vi "gyro-V2.vi"() -> ()   [LabVIEW 2016]
uses:
  lorentzian.ctl
  circle corners.ctl
  <vilib>/event_ctls.llb/eventvkey.ctl
  peak -- parameters -- complex fit.ctl
  wavepacket.ctl
  filter method control.ctl
  cursor winow.ctl
  parameters -- scan monitor control.ctl
  pid -- parameters.ctl
  agregator -- action.ctl
  plot refs -- filter related.ctl
  MFLI controller action.ctl
  cursor window action.ctl
  sweep parameters.ctl
  cursor action.ctl
  KM_file -- read-write control.ctl
  linear interpolation - real.vi
  linear interpolation iiii- complex.vi
  aggregator - v - real - atomic.vi
  Q - not nan -- real.vi
  filter - complex - four.vi
  linear interp iiii- complex - z-omega.vi
  peak -- PM find lorenzian - V3.vi
  tale of three indices.vi
  filter -- window span logic.vi
  linear interp iiii- complex - z-omega - divide.vi
  containing bix.vi
  <vilib>/Analysis/baseanly.llb/A x B.vi
  <vilib>/Analysis/baseanly.llb/Complex A x B.vi
  line -- complex.vi
  Q -- check range -- i -- integer.vi
  peak -- guess at omega -- dzdomega V2.vi
  command stack.vi
  tale of three indices -- check state.vi
  Q - not nan -- integer.vi
  peak -- z center from mult phase points.vi
  peak -- estimate for lorentzian.vi
  peak -- fake phase around center.vi
  peak -- get weights.vi
  peak -- four corner circle transformation logic.vi
  peak - fit phase around center - V2.vi
  array - generate range.vi
  circle center from three points.vi
  <vilib>/Utility/error.llb/Clear Errors.vi
  peak -- fit function -- minus arctan.vi
  <vilib>/Analysis/Matrix/Numeric/Conversions/Array To Matrix.vi
  <vilib>/Analysis/Matrix/Numeric/Conversions/Array To Matrix - RA2.vi
  <vilib>/Analysis/baseanly.llb/Inverse Matrix.vi
  <vilib>/Analysis/baseanly.llb/Real Inverse Matrix.vi
  <vilib>/gmath/NumericalOptimization/Nonlinear Curve Fit.vi
  <vilib>/gmath/NumericalOptimization/Nonlinear Curve Fit LM.vi
  KM_filter pipe - plot staff - more - V3.vi
  four-corner circle transformation.ctl
panel:
  in  "all":enum32{"all", "other"}(tab)
  out "angle (deg)":dbl=1994442.711851292 format="%#11_11f"
  out "Temperature (K)":dbl=1994442.711851292 format="%#11_11f"
  out "Field (T)":dbl=1994442.711851292 format="%#11_11f"
  out "Plot: circle sweep window":cluster{"all rows":dbl[], "all rows":dbl[]}[](graph)=[{"all rows"=[1907168.346185415, 1965249.3711735276, 1976970.6285003964, 1982011.816659579, 1984821.3372776513, 1986615.362944235, 1987862.2368974418, 1988780.6904674931, 1989486.5864630162, 1990047.0317770669, 1990503.5833778584, 1990883.3521453317, 1991204.7790270294, 1991480.8449781418, 1991720.9531195113, 1991932.0825617604, 1992119.5227900057, 1992287.356339517, 1992438.7849751213, 1992576.3555406206, 1992702.1197279515, 1992817.749276128, 1992924.6204638672, 1993023.8770414377, 1993116.4777602106, 1993203.2327275807, 1993284.831541473, 1993361.8652934371, 1993434.843950368, 1993504.210209025, 1993570.3506361335, 1993633.604695191, 1993694.2721197682, 1993752.6189752219, 1993808.8826808098, 1993863.276194716, 1993915.991524844, 1993967.2026947618, 1994017.0682615843, 1994065.733471473, 1994113.3321128746, 1994159.9881239824, 1994205.8169966259, 1994250.9270102703, 1994295.4203281004, 1994339.393978848, 1994382.940745254, 1994426.14997686, 1994469.108344603, 1994511.9005478774, 1994554.6099904731, 1994597.3194328558, 1994640.1116363432, 1994683.0700038732, 1994726.2792356922, 1994769.8260018853, 1994813.7996526328, 1994858.2929704627, 1994903.4029841074, 1994949.2318567508, 1994995.887868072, 1995043.4865092603, 1995092.151719149, 1995142.0172861845, 1995193.2284558893, 1995245.9437862302, 1995300.3372999234, 1995356.6010057244, 1995414.9478611783, 1995475.6152855423, 1995538.8693448128, 1995605.0097717082, 1995674.3760305785, 1995747.354687296, 1995824.3884394732, 1995905.9872531525, 1995992.7422207356, 1996085.3429392956, 1996184.599517079, 1996291.4707048186, 1996407.1002529948, 1996532.8644403256, 1996670.435005825, 1996821.8636414292, 1996989.6971907276, 1997177.137419186, 1997388.266861222, 1997628.3750028044, 1997904.440953917, 1998225.8678354016, 1998605.636603088, 1999062.1882036664, 1999622.63351793, 2000328.5295134531, 2001246.9830832912, 2002493.8570367112, 2004287.882703082, 2007097.4033211542, 2012138.5914805501], "all rows"=[2.3267514059577948e-05, 2.4909528000811873e-05, 2.493131520279196e-05, 2.4976654073748857e-05, 2.5405139290521606e-05, 2.4883129570955604e-05, 2.512681802676727e-05, 2.5324670293110625e-05, 2.5110327803608353e-05, 2.489327033666908e-05, 2.472882726006047e-05, 2.4998415038301484e-05, 2.500505012592314e-05, 2.5078583497907004e-05, 2.4694152114450753e-05, 2.5044541628387363e-05, 2.4861233245129487e-05, 2.488726435100131e-05, 2.4957802482118494e-05, 2.46934049440733e-05, 2.441914511482881e-05, 2.382274155491927e-05, 2.414210352196834e-05, 2.399883643454102e-05, 2.350820965974361e-05, 2.3707949231948613e-05, 2.3627483216063482e-05, 2.3077478161397138e-05, 2.2546323505750814e-05, 2.2846480868509143e-05, 2.1846370956842606e-05, 2.1881777768895366e-05, 2.139614922402918e-05, 2.0837511459423164e-05, 1.9785950548811776e-05, 1.93704111172701e-05, 1.8487665392770513e-05, 1.6839358643082255e-05, 1.5292283044198602e-05, 1.2966042313988014e-05, 1.0214084415601758e-05, 6.819459217031084e-06, 2.984185965144213e-06, -2.279309128145807e-06, -8.090223100581805e-06, -1.48470398632458e-05, -2.0660352771378924e-05, -2.415896464694272e-05, -2.3951911391833105e-05, -2.0449413395479307e-05, -1.4517394017242558e-05, -8.22062728919662e-06, -2.901640633132837e-06, 1.3769986310330702e-06, 6.276775597236554e-06, 9.235612629622917e-06, 1.1399920727988725e-05, 1.4010038497218408e-05, 1.5579325867362877e-05, 1.7058951599602477e-05, 1.8183437054619616e-05, 1.9258252077928204e-05, 1.9764283204170766e-05, 2.046705746914132e-05, 2.0724465117988968e-05, 2.1028962986076503e-05, 2.2105881774023284e-05, 2.195269216857454e-05, 2.2944142536568783e-05, 2.2594225296326463e-05, 2.2991647784206674e-05, 2.3061333198931392e-05, 2.2895663522589002e-05, 2.3522359385112018e-05, 2.3758774110465428e-05, 2.4074391877354853e-05, 2.369724972829126e-05, 2.4196489534957747e-05, 2.4788286637432465e-05, 2.437100659110085e-05, 2.4436145178907698e-05, 2.4630974178041407e-05, 2.5085569212968363e-05, 2.4928911496653477e-05, 2.4997082296247526e-05, 2.481615794105754e-05, 2.4256112896251368e-05, 2.519658215377437e-05, 2.5386526220959067e-05, 2.5195390736045592e-05, 2.491297345208157e-05, 2.490013440547585e-05, 2.473084575305942e-05, 2.5244618113013167e-05, 2.519002518212992e-05, 2.5127560426703364e-05, 2.5077375979938654e-05, 2.429082024234024e-05, 2.478161100105928e-05]}, {"all rows"=[1907168.346185415, 1965249.3711735276, 1976970.6285003964, 1982011.816659579, 1984821.3372776513, 1986615.362944235, 1987862.2368974418, 1988780.6904674931, 1989486.5864630162, 1990047.0317770669, 1990503.5833778584, 1990883.3521453317, 1991204.7790270294, 1991480.8449781418, 1991720.9531195113, 1991932.0825617604, 1992119.5227900057, 1992287.356339517, 1992438.7849751213, 1992576.3555406206, 1992702.1197279515, 1992817.749276128, 1992924.6204638672, 1993023.8770414377, 1993116.4777602106, 1993203.2327275807, 1993284.831541473, 1993361.8652934371, 1993434.843950368, 1993504.210209025, 1993570.3506361335, 1993633.604695191, 1993694.2721197682, 1993752.6189752219, 1993808.8826808098, 1993863.276194716, 1993915.991524844, 1993967.2026947618, 1994017.0682615843, 1994065.733471473, 1994113.3321128746, 1994159.9881239824, 1994205.8169966259, 1994250.9270102703, 1994295.4203281004, 1994339.393978848, 1994382.940745254, 1994426.14997686, 1994469.108344603, 1994511.9005478774, 1994554.6099904731, 1994597.3194328558, 1994640.1116363432, 1994683.0700038732, 1994726.2792356922, 1994769.8260018853, 1994813.7996526328, 1994858.2929704627, 1994903.4029841074, 1994949.2318567508, 1994995.887868072, 1995043.4865092603, 1995092.151719149, 1995142.0172861845, 1995193.2284558893, 1995245.9437862302, 1995300.3372999234, 1995356.6010057244, 1995414.9478611783, 1995475.6152855423, 1995538.8693448128, 1995605.0097717082, 1995674.3760305785, 1995747.354687296, 1995824.3884394732, 1995905.9872531525, 1995992.7422207356, 1996085.3429392956, 1996184.599517079, 1996291.4707048186, 1996407.1002529948, 1996532.8644403256, 1996670.435005825, 1996821.8636414292, 1996989.6971907276, 1997177.137419186, 1997388.266861222, 1997628.3750028044, 1997904.440953917, 1998225.8678354016, 1998605.636603088, 1999062.1882036664, 1999622.63351793, 2000328.5295134531, 2001246.9830832912, 2002493.8570367112, 2004287.882703082, 2007097.4033211542, 2012138.5914805501], "all rows"=[0.0007497899281750819, 0.0007493263849847805, 0.0007496174170895291, 0.0007494851506398698, 0.0007499570558175639, 0.000749671639118597, 0.0007497804737566186, 0.0007503679858101448, 0.0007502255702464996, 0.0007506115096857297, 0.0007515632145252575, 0.0007513210836185486, 0.000751689059960851, 0.0007518588196943513, 0.0007527186541816263, 0.0007526931913545811, 0.0007527422720404769, 0.0007539103456144731, 0.0007536834592494241, 0.0007546041049378904, 0.0007547662426987134, 0.0007552009676527804, 0.0007555408747181414, 0.0007557323978014151, 0.0007559722204108125, 0.0007566726869747769, 0.0007571410924374308, 0.0007579726495372601, 0.000759089640032601, 0.0007591964764519996, 0.0007603545201730438, 0.0007613896552614546, 0.0007619913617632369, 0.00076253003105663, 0.000764456902958887, 0.0007649733360325073, 0.0007661060188946903, 0.0007671367407285413, 0.0007682815906014038, 0.0007701434771662825, 0.0007711845222352289, 0.000772082315124377, 0.0007735724769726575, 0.0007734071418235152, 0.0007718988278495682, 0.000767734527120139, 0.0007624145887610245, 0.0007536607072256797, 0.0007439809384794281, 0.0007355586616525682, 0.0007285883199347894, 0.0007254664047683276, 0.0007241688059595365, 0.000724465102246322, 0.0007245410947808251, 0.0007259112698918029, 0.0007267781228909235, 0.000728309312323785, 0.0007294235431188013, 0.0007307315832311114, 0.0007319223295202645, 0.0007324354566780247, 0.0007333411154286644, 0.0007339010340567747, 0.0007349364953241133, 0.000735803180165176, 0.0007365826661086842, 0.0007370666351362634, 0.000738127734544367, 0.0007379654494961671, 0.0007395610917658905, 0.0007392509647770023, 0.0007392496570797655, 0.0007401551101051218, 0.0007409229758497907, 0.0007408003808736765, 0.0007419127553707, 0.0007416263905465133, 0.0007423997071167373, 0.0007423726956851667, 0.0007433577459097762, 0.0007429029540941432, 0.0007433307970902484, 0.0007437865358384905, 0.0007440816556151765, 0.000744689260767696, 0.0007446534419087711, 0.0007455103199150154, 0.0007450821310619119, 0.0007456887582739535, 0.0007453899491571836, 0.0007459573174257771, 0.0007462436035376812, 0.0007469393026418149, 0.0007468684747063853, 0.0007468887240373331, 0.000747052914876855, 0.0007474931306089232, 0.0007475443788641105]}]
  out "Plot: frequency shift vs T":cluster{dbl[], dbl[]}(graph)
  in  "MFLI mode":enum32{"circles sweep", "read", "circle PLL"}(tab)=enum."circle PLL"
  out "fit is fine":bool=TRUE
  in  "gamma factor":dbl=2.0
  in  "Auto-update sweep window!":bool
  in  "scan type":enum16{"linear", "arctan"}(ring)=enum."arctan"
  in  "N":i64=100
  out "sweep time (sec)":dbl=5.013347714149859
  in  "control sweep!":bool=TRUE
  out "circle frequency (Hz)":dbl=1994442.711851292 format="%#11_11f"
  out "circle gamma (Hz)":dbl=1994442.711851292 format="%#11_11f"
  out "circle phase (rad)":dbl=1994442.711851292 format="%#11_11f"
  out "circle Q":dbl=1994442.711851292 format="%#11_11f"
  out "read Voltage (V)":cdb=-2.4433028888091597e-05+0.0007504399568625844i format="%#10_10f"
  in  "read !":bool=TRUE
  out "read freq (Hz)":dbl=1994442.711851292 format="%#11_11f"
  out "read Voltage X (V)":dbl=1994442.711851292 format="%#11_11f"
  out "read Voltage Y (V)":dbl=1994442.711851292 format="%#11_11f"
  in  "reqested size":i64=30
  in  "refresh":bool=TRUE
  in  "PID parameters":T1={"P (sec)"=60.0, "I (sec)"=10.0}
  in  "MFLI Address":string="DEV3523"
  in  "save data":enum32{"save"}(tab)
  in  "save data ?":bool
  in  "File name":string="lowT_turnonfield.dat"
  in  "Save folder":path=path "D:/data/TestFolder/1_test"
  out "left freq (Hz)":dbl=5.013347714149859
  out "right freq (Hz)":dbl=5.013347714149859
  in  "horisontal axis":enum16{"Time", "temperature", "field", "angle"}(ring)=enum."angle"
  in  "vertical axis":T2(ring)=enum."background"
  out "center freq (Hz)":dbl=5.013347714149859
  out "window  (Hz)":dbl=5.013347714149859
  in  "delay (msec)":i64=100
  in  "talk to MFLI !":bool=TRUE
  in  "plot frequency shift":enum32{"plot"}(tab)
  in  "Plot frequency shift":bool=TRUE
  in  "aggregate every # sec":dbl=1.0
  in  "plot length (min)":dbl=100.0
  out "Plot: frequency shift vs T 4":cluster{dbl[], dbl[]}(graph)
  out "Plot: frequency shift vs T 5":cluster{i32[], "Array":dbl[]}(graph)
  out "Plot: frequency shift vs T 2":cluster{dbl[], dbl[]}(graph)={[-1.2847105611270713e-06, -8.96090687489996e-07, -1.1878113186140714e-06, -1.0577364834927965e-06, -1.5485833177118755e-06, -1.2397929198806674e-06, -1.3595641386431873e-06, -1.95544238796184e-06, -1.8034552812236216e-06, -2.179156763955588e-06, -3.122427320687229e-06, -2.8927681404839808e-06, -3.2606669096266067e-06, -3.4335859766558394e-06, -4.275106687632253e-06, -4.265556221219542e-06, -4.306275487364196e-06, -5.474328117771029e-06, -5.250873166830706e-06, -6.158584714145268e-06, -6.308121182987117e-06, -6.715358985348123e-06, -7.0693959466281e-06, -7.254226550276167e-06, -7.471558204043555e-06, -8.180360377818478e-06, -8.644635949920024e-06, -9.450401470204308e-06, -1.0542161519072343e-05, -1.0662496796273006e-05, -1.1774006071250966e-05, -1.2809682001462881e-05, -1.3388752026600543e-05, -1.3901539528835397e-05, -1.577875366340369e-05, -1.6275815692673765e-05, -1.7367311318108792e-05, -1.8322241284696204e-05, -1.939577161026033e-05, -2.115027501101159e-05, -2.206547957836183e-05, -2.280844162782534e-05, -2.4123185115153962e-05, -2.3719380386582883e-05, -2.1949158634554497e-05, -1.7482795415692865e-05, -1.190476009852551e-05, -3.0012581586913445e-06, 6.6591691413936944e-06, 1.4913986718231652e-05, 2.1608211101800334e-05, 2.4441429222012755e-05, 2.5496538170609067e-05, 2.5006558977858244e-05, 2.47084954682896e-05, 2.3205579756867926e-05, 2.2241491423599197e-05, 2.059353741490501e-05, 1.940930308820722e-05, 1.8035523877789703e-05, 1.6795019444131693e-05, 1.6233689318685545e-05, 1.530601912625958e-05, 1.471481346136583e-05, 1.3668746476334144e-05, 1.278914735524648e-05, 1.1961636965375277e-05, 1.148511101983816e-05, 1.038015177533868e-05, 1.055813470630652e-05, 8.946114686992878e-06, 9.252763324432675e-06, 9.261580911233215e-06, 8.32864546005932e-06, 7.550850612980853e-06, 7.659009848135973e-06, 6.564878336519785e-06, 6.828313841636074e-06, 6.028961228097367e-06, 6.074863784114649e-06, 5.087873216594783e-06, 5.533364081213274e-06, 5.085350335296872e-06, 4.637182878582281e-06, 4.339275810721466e-06, 3.7404983334720106e-06, 3.8016720277973716e-06, 2.9030355925414103e-06, 3.3221723271601737e-06, 2.724834743267001e-06, 3.0361409970562057e-06, 2.469938271454002e-06, 2.1916218680781524e-06, 1.473344438791089e-06, 1.5465747082434236e-06, 1.5291782659004455e-06, 1.3674315612440997e-06, 9.633298642757269e-07, 8.898825337811226e-07], [-5.351696133733621e-06, -3.690354306686691e-06, -3.6817845026587138e-06, -3.6304954766072717e-06, -3.2238464103788782e-06, -3.732378935963822e-06, -3.493875482979771e-06, -3.3228636578776652e-06, -3.5305288089255853e-06, -3.7648610315931326e-06, -3.97228399037134e-06, -3.69199555481082e-06, -3.702050829314118e-06, -3.6362897452965515e-06, -4.059309516809881e-06, -3.708125867376757e-06, -3.8934710007503085e-06, -3.920425505771773e-06, -3.8396731962881915e-06, -4.145539651931423e-06, -4.426868555366925e-06, -5.042368648209767e-06, -4.738746005563639e-06, -4.890549160081816e-06, -5.391544637503511e-06, -5.223768648790353e-06, -5.325388776256424e-06, -5.912529897926599e-06, -6.493781160800396e-06, -6.198776272723992e-06, -7.250361850269486e-06, -7.26192304305288e-06, -7.774332746184141e-06, -8.356818571969059e-06, -9.494659847987037e-06, -9.933186332652295e-06, -1.0866378585117719e-05, -1.2559721845876861e-05, -1.4157112461896858e-05, -1.656537642835046e-05, -1.936170396817286e-05, -2.2793543082063973e-05, -2.6692434310764325e-05, -3.194302075894453e-05, -3.767957435737811e-05, -4.424063928058543e-05, -4.980677556288027e-05, -5.2904900834404434e-05, -5.2259193151987076e-05, -4.837844245967899e-05, -4.2136497452806694e-05, -3.570466251887759e-05, -3.0332314166196737e-05, -2.6071508393447144e-05, -2.1180215381563472e-05, -1.8286542839044908e-05, -1.61637622680976e-05, -1.3625750559341328e-05, -1.2108594610162641e-05, -1.0689795144437375e-05, -9.62045281676502e-06, -8.570007528029048e-06, -8.105558082533694e-06, -7.428892434368157e-06, -7.218695867625404e-06, -6.953805415589833e-06, -5.913334865014344e-06, -6.088309429175753e-06, -5.145987374849902e-06, -5.488187006895521e-06, -5.163517414643828e-06, -5.079842929772351e-06, -5.245282954840261e-06, -4.660283528196666e-06, -4.4589258860321075e-06, -4.13807438954911e-06, -4.565262237593832e-06, -4.053552425555827e-06, -3.4974249873645082e-06, -3.913051273651945e-06, -3.89264048603008e-06, -3.6773922014571442e-06, -3.2426624479706957e-06, -3.419821634783878e-06, -3.3651012599037013e-06, -3.573387544637086e-06, -4.131232704147514e-06, -3.2305802189117116e-06, -3.021417984572191e-06, -3.2398605602097806e-06, -3.508439835095558e-06, -3.546989372643574e-06, -3.729083758383661e-06, -3.2473817592994867e-06, -3.29870731020323e-06, -3.3620259083252726e-06, -3.419602935105049e-06, -4.225308611898116e-06, -3.737346070152369e-06]}
  out "Plot: frequency shift vs T 3":cluster{i32[], dbl[]}(graph)={[0, 1, 2, 3, 4, 5, 6, 7, 8, 9, 10, 11, 12, 13, 14, 15, 16, 17, 18, 19, 20, 21, 22, 23, 24, 25, 26, 27, 28, 29, 30, 31, 32, 33, 34, 35, 36, 37, 38, 39, 40, 41, 42, 43, 44, 45, 46, 47, 48, 49, 50, 51, 52, 53, 54, 55, 56, 57, 58, 59, 60, 61, 62, 63, 64, 65, 66, 67, 68, 69, 70, 71, 72, 73, 74, 75, 76, 77, 78, 79, 80, 81, 82, 83, 84, 85, 86, 87, 88, 89, 90, 91, 92, 93, 94, 95, 96, 97, 98], [-0.23559860043831193, -0.23820939062512414, -0.3120762913359678, -0.2835001183703665, -0.44780658796424877, -0.32070526654251785, -0.37109881260414546, -0.5319066481282504, -0.4722639722623221, -0.524696373474268, -0.6661788735811576, -0.6646137200418041, -0.7220903993361305, -0.7567345405074919, -0.8112846755002696, -0.8551933851256885, -0.8356992634466227, -0.9493152294582043, -0.9394070576242828, -0.9783311582294316, -0.9588814811243913, -0.9267379794474269, -0.9802698763137818, -0.9776201855738149, -0.9457143265769079, -1.0024951473096775, -1.0186705422504727, -1.0117383851591542, -1.0187082032726575, -1.0441935724590885, -1.0188444902666154, -1.0550639642963695, -1.0447176937736993, -1.0295365240674577, -1.0291006014399389, -1.0228351916589804, -1.0117082035896368, -0.9698748205564658, -0.9402791409053437, -0.9063694667492768, -0.8505714661765986, -0.7857248716608289, -0.7348809545553663, -0.6387178563870073, -0.5274684440579174, -0.37634000181515215, -0.2346170964234171, -0.05666856473380277, 0.12674275046362427, 0.29903345155814187, 0.4738466551438263, 0.6002776366427447, 0.6989959497442624, 0.7645517375308588, 0.8621349432337582, 0.9034008935958421, 0.9423491262817814, 0.9862736125756424, 1.0130206638602015, 1.035756014091886, 1.050605066301123, 1.0850669404773998, 1.083776083480046, 1.1032698129216518, 1.0849090392836143, 1.0727819505921015, 1.1116722316992618, 1.0833561407376393, 1.1105523962821076, 1.0914293641785555, 1.0473253514157124, 1.0687148941515687, 1.0554881441119783, 1.060651558581904, 1.0373768137660564, 1.0754397797680961, 0.9631595802552361, 1.0350672662925295, 1.0451346582720782, 0.9985529870514799, 0.9177123734459048, 0.984236082337904, 1.0031536192825101, 0.9353574049208152, 0.9111749823496003, 0.8082426158031351, 0.7438785320162125, 0.7320472832267922, 0.8327734332640132, 0.6992660900455262, 0.7133566540037093, 0.6082706202737593, 0.5313341296869087, 0.42592845813496805, 0.438412524592966, 0.42687019592046394, 0.38040311101033075, 0.22415893312212232, 0.2337528615998219]}
  in  "aggregator action":T3
  in  "Tab : everything":T4(tab)
  in  "Tab :  Fit controls":enum32{"complex plane", "complex plane 2"}(tab)
  in  "Plot: fragment - filter":cluster{dbl[], dbl[]}[](graph)=[{[1993203.2327275807, 1993284.831541473, 1993361.8652934371, 1993434.843950368, 1993504.210209025, 1993570.3506361335, 1993633.604695191, 1993694.2721197682, 1993752.6189752219, 1993808.8826808098, 1993863.276194716, 1993915.991524844, 1993967.2026947618, 1994017.0682615843, 1994065.733471473, 1994113.3321128746, 1994159.9881239824, 1994205.8169966259, 1994250.9270102703, 1994295.4203281004, 1994339.393978848, 1994382.940745254, 1994426.14997686, 1994469.108344603, 1994511.9005478774, 1994554.6099904731, 1994597.3194328558, 1994640.1116363432, 1994683.0700038732, 1994726.2792356922, 1994769.8260018853, 1994813.7996526328, 1994858.2929704627, 1994903.4029841074, 1994949.2318567508, 1994995.887868072, 1995043.4865092603, 1995092.151719149, 1995142.0172861845, 1995193.2284558893, 1995245.9437862302, 1995300.3372999234, 1995356.6010057244, 1995414.9478611783, 1995475.6152855423, 1995538.8693448128, 1995605.0097717082, 1995674.3760305785, 1995747.354687296, 1995824.3884394732], [9.455717362020653e-06, 9.263582241804865e-06, 8.52759457850524e-06, 7.740364677546865e-06, 8.005458949117915e-06, 6.753398338983944e-06, 6.535604078552307e-06, 5.918040237333932e-06, 5.245020481003143e-06, 3.755789941302106e-06, 3.2269748570983087e-06, 2.0949209317757097e-06, 2.4519872491622085e-07, -1.534140163814164e-06, -4.2438303816745295e-06, -7.166478100183732e-06, -1.0677544171656513e-05, -1.4760273923502824e-05, -1.9824969533744665e-05, -2.5093478470951677e-05, -3.0632464975632874e-05, -3.497487811463608e-05, -3.6235876983368224e-05, -3.36772947343491e-05, -2.8228816651746977e-05, -2.0777647734436005e-05, -1.3910103678541439e-05, -8.43525134960928e-06, -4.357648418026914e-06, 3.760454193714239e-07, 2.912024620069612e-06, 4.8000022609253e-06, 6.958545722235614e-06, 8.209168228008998e-06, 9.325622141942974e-06, 1.0126202042482199e-05, 1.1043659661485757e-05, 1.1313852699535082e-05, 1.1859077501615568e-05, 1.1856518332760824e-05, 1.1940741091037332e-05, 1.279536034721289e-05, 1.2528901030775737e-05, 1.323203158525885e-05, 1.2932182108980333e-05, 1.292897378518709e-05, 1.307210006660186e-05, 1.291173860957817e-05, 1.3299012272770984e-05, 1.3341272458076386e-05]}, {[1993203.2327275807, 1993284.831541473, 1993361.8652934371, 1993434.843950368, 1993504.210209025, 1993570.3506361335, 1993633.604695191, 1993694.2721197682, 1993752.6189752219, 1993808.8826808098, 1993863.276194716, 1993915.991524844, 1993967.2026947618, 1994017.0682615843, 1994065.733471473, 1994113.3321128746, 1994159.9881239824, 1994205.8169966259, 1994250.9270102703, 1994295.4203281004, 1994339.393978848, 1994382.940745254, 1994426.14997686, 1994469.108344603, 1994511.9005478774, 1994554.6099904731, 1994597.3194328558, 1994640.1116363432, 1994683.0700038732, 1994726.2792356922, 1994769.8260018853, 1994813.7996526328, 1994858.2929704627, 1994903.4029841074, 1994949.2318567508, 1994995.887868072, 1995043.4865092603, 1995092.151719149, 1995142.0172861845, 1995193.2284558893, 1995245.9437862302, 1995300.3372999234, 1995356.6010057244, 1995414.9478611783, 1995475.6152855423, 1995538.8693448128, 1995605.0097717082, 1995674.3760305785, 1995747.354687296, 1995824.3884394732], [1.1676838483358423e-05, 1.211153671516539e-05, 1.2784080341933105e-05, 1.3738052101438482e-05, 1.3914782093539839e-05, 1.479434410034474e-05, 1.580692691361086e-05, 1.6272223270673325e-05, 1.6658597658122914e-05, 1.8271299762063677e-05, 1.867096305211354e-05, 1.9554515195774e-05, 2.0152704461220897e-05, 2.0886241957949105e-05, 2.2125433806937156e-05, 2.246481180204127e-05, 2.2508713423066363e-05, 2.3019811284633563e-05, 2.1577391552299383e-05, 1.869910285628129e-05, 1.3014421525696338e-05, 6.438723901652362e-06, -2.903685254649011e-06, -1.2241482152545503e-05, -1.955696749161405e-05, -2.487247304913933e-05, -2.636661634024566e-05, -2.632955298439642e-05, -2.5000004273451264e-05, -2.3732829527169034e-05, -2.1683218365853275e-05, -2.031529874308107e-05, -1.8194462593306728e-05, -1.6731548903880468e-05, -1.5102502587479615e-05, -1.367372125832896e-05, -1.2914248854818922e-05, -1.1912609700469291e-05, -1.1198375528221814e-05, -1.013140215250033e-05, -9.216651862865997e-06, -8.198330529035862e-06, -7.76625124515689e-06, -6.495616282067166e-06, -6.738245224000234e-06, -5.093858227743186e-06, -5.377670972049305e-06, -5.419292538967123e-06, -4.3884618084261736e-06, -3.586137808449955e-06]}, {[1993203.2327275807, 1993284.831541473, 1993361.8652934371, 1993434.843950368, 1993504.210209025, 1993570.3506361335, 1993633.604695191, 1993694.2721197682, 1993752.6189752219, 1993808.8826808098, 1993863.276194716, 1993915.991524844, 1993967.2026947618, 1994017.0682615843, 1994065.733471473, 1994113.3321128746, 1994159.9881239824, 1994205.8169966259, 1994250.9270102703, 1994295.4203281004, 1994339.393978848, 1994382.940745254, 1994426.14997686, 1994469.108344603, 1994511.9005478774, 1994554.6099904731, 1994597.3194328558, 1994640.1116363432, 1994683.0700038732, 1994726.2792356922, 1994769.8260018853, 1994813.7996526328, 1994858.2929704627, 1994903.4029841074, 1994949.2318567508, 1994995.887868072, 1995043.4865092603, 1995092.151719149, 1995142.0172861845, 1995193.2284558893, 1995245.9437862302, 1995300.3372999234, 1995356.6010057244, 1995414.9478611783, 1995475.6152855423, 1995538.8693448128, 1995605.0097717082, 1995674.3760305785, 1995747.354687296, 1995824.3884394732], [9.923052351053618e-06, 9.211940146396975e-06, 8.540611255951826e-06, 7.904621452332785e-06, 7.300112749699984e-06, 6.723716320703672e-06, 6.0695317303198386e-06, 5.3240195905895175e-06, 4.427645284648154e-06, 3.401618861190508e-06, 2.0725847518192263e-06, 5.196735378420159e-07, -1.3800541486556074e-06, -3.6542833253257687e-06, -6.402962205838908e-06, -9.572283420893726e-06, -1.3227365822979675e-05, -1.71413125132564e-05, -2.084928529107787e-05, -2.3868544063595353e-05, -2.5803250617472023e-05, -2.644370764553595e-05, -2.5903162538725086e-05, -2.4395324243348082e-05, -2.2096278962280914e-05, -1.896182432917072e-05, -1.5307214832257182e-05, -1.1330273951392744e-05, -7.227890185441405e-06, -3.3844339408855624e-06, -1.9505592320177843e-09, 2.7661251747950676e-06, 5.009266389085727e-06, 6.774057725731099e-06, 8.220053731840045e-06, 9.247837511129577e-06, 1.0049078401514694e-05, 1.0777196493458952e-05, 1.127760287104988e-05, 1.1747021058090037e-05, 1.2074430024453888e-05, 1.2326346135779358e-05, 1.2514335396813481e-05, 1.2598423842010029e-05, 1.2793124553480302e-05, 1.2925185979961812e-05, 1.3113342114628652e-05, 1.3280752244100232e-05, 1.2513826667888714e-05, 1.2598423842010029e-05]}, {[1993203.2327275807, 1993284.831541473, 1993361.8652934371, 1993434.843950368, 1993504.210209025, 1993570.3506361335, 1993633.604695191, 1993694.2721197682, 1993752.6189752219, 1993808.8826808098, 1993863.276194716, 1993915.991524844, 1993967.2026947618, 1994017.0682615843, 1994065.733471473, 1994113.3321128746, 1994159.9881239824, 1994205.8169966259, 1994250.9270102703, 1994295.4203281004, 1994339.393978848, 1994382.940745254, 1994426.14997686, 1994469.108344603, 1994511.9005478774, 1994554.6099904731, 1994597.3194328558, 1994640.1116363432, 1994683.0700038732, 1994726.2792356922, 1994769.8260018853, 1994813.7996526328, 1994858.2929704627, 1994903.4029841074, 1994949.2318567508, 1994995.887868072, 1995043.4865092603, 1995092.151719149, 1995142.0172861845, 1995193.2284558893, 1995245.9437862302, 1995300.3372999234, 1995356.6010057244, 1995414.9478611783, 1995475.6152855423, 1995538.8693448128, 1995605.0097717082, 1995674.3760305785, 1995747.354687296, 1995824.3884394732], [1.1258927442316528e-05, 1.2107275955839959e-05, 1.2908163442464435e-05, 1.3666891813295672e-05, 1.4388063600154742e-05, 1.507569777453331e-05, 1.5785838752451718e-05, 1.6534908519376068e-05, 1.72686726167956e-05, 1.799048342600788e-05, 1.8811756958989244e-05, 1.9566286956450066e-05, 2.0211580071947433e-05, 2.0847841086689058e-05, 2.122335539351363e-05, 2.1092008381884776e-05, 2.0192823855609292e-05, 1.8426193347819905e-05, 1.550471844416874e-05, 1.1492216084211813e-05, 6.688026106541281e-06, 1.4618706089641872e-06, -3.643762023882996e-06, -8.462295366709863e-06, -1.2710582901210136e-05, -1.6331394127849216e-05, -1.907362379819513e-05, -2.1016058143101085e-05, -2.1923521137337555e-05, -2.1940249246234295e-05, -2.1236922596965e-05, -2.0018286409807475e-05, -1.866495934178386e-05, -1.726223003459208e-05, -1.5940526359288458e-05, -1.4646988709753693e-05, -1.3455916413347887e-05, -1.229922237489627e-05, -1.1303069566718817e-05, -1.030846829590753e-05, -9.512361367064947e-06, -8.662014716093488e-06, -7.941683322124457e-06, -7.479348644755681e-06, -6.683144776467428e-06, -6.078308409569257e-06, -5.18055455265303e-06, -4.394587341134809e-06, -7.995195969048528e-06, -7.479348644755681e-06]}]
  in  "scale gauge: Plot: complex plane - filter":dbl(slide)=9.999999999999991e-05 min=0.0 max=0.3 step=1e-05 scale=0.0001..0.3 scale format="%#_5g"
  in  "Plot: complex plane - filter":cluster{dbl[], dbl[]}[](graph)=[{[2.3707949231948613e-05, 2.3627483216063482e-05, 2.3077478161397138e-05, 2.2546323505750814e-05, 2.2846480868509143e-05, 2.1846370956842606e-05, 2.1881777768895366e-05, 2.139614922402918e-05, 2.0837511459423164e-05, 1.9785950548811776e-05, 1.93704111172701e-05, 1.8487665392770513e-05, 1.6839358643082255e-05, 1.5292283044198602e-05, 1.2966042313988014e-05, 1.0214084415601758e-05, 6.819459217031084e-06, 2.9841859651442124e-06, -2.279309128145807e-06, -8.090223100581807e-06, -1.48470398632458e-05, -2.066035277137892e-05, -2.415896464694272e-05, -2.39519113918331e-05, -2.0449413395479304e-05, -1.451739401724256e-05, -8.220627289196623e-06, -2.9016406331328374e-06, 1.3769986310330693e-06, 6.276775597236554e-06, 9.235612629622917e-06, 1.1399920727988725e-05, 1.4010038497218408e-05, 1.5579325867362877e-05, 1.7058951599602477e-05, 1.8183437054619616e-05, 1.9258252077928204e-05, 1.9764283204170766e-05, 2.046705746914132e-05, 2.0724465117988968e-05, 2.1028962986076503e-05, 2.2105881774023284e-05, 2.195269216857454e-05, 2.2944142536568783e-05, 2.2594225296326463e-05, 2.2991647784206674e-05, 2.3061333198931392e-05, 2.2895663522589002e-05, 2.3522359385112018e-05, 2.3758774110465428e-05], [0.0007566726869747769, 0.0007571410924374308, 0.0007579726495372601, 0.000759089640032601, 0.0007591964764519996, 0.0007603545201730438, 0.0007613896552614546, 0.0007619913617632369, 0.00076253003105663, 0.000764456902958887, 0.0007649733360325073, 0.0007661060188946903, 0.0007671367407285413, 0.0007682815906014038, 0.0007701434771662825, 0.0007711845222352289, 0.000772082315124377, 0.0007735724769726575, 0.0007734071418235152, 0.0007718988278495682, 0.000767734527120139, 0.0007624145887610245, 0.0007536607072256797, 0.0007439809384794281, 0.0007355586616525682, 0.0007285883199347894, 0.0007254664047683276, 0.0007241688059595365, 0.000724465102246322, 0.0007245410947808251, 0.0007259112698918029, 0.0007267781228909235, 0.000728309312323785, 0.0007294235431188013, 0.0007307315832311114, 0.0007319223295202645, 0.0007324354566780247, 0.0007333411154286644, 0.0007339010340567747, 0.0007349364953241133, 0.000735803180165176, 0.0007365826661086842, 0.0007370666351362634, 0.000738127734544367, 0.0007379654494961671, 0.0007395610917658905, 0.0007392509647770023, 0.0007392496570797655, 0.0007401551101051218, 0.0007409229758497907]}, {[2.4059415521428895e-05, 2.357635867336631e-05, 2.3120326537076183e-05, 2.2688300159348305e-05, 2.2277658819475025e-05, 2.188611408096243e-05, 2.1424606161526664e-05, 2.0884003468308606e-05, 2.0193354223370333e-05, 1.9374046225661016e-05, 1.8285083420554144e-05, 1.696272915357647e-05, 1.5277396401376255e-05, 1.322664151216894e-05, 1.0652214759659831e-05, 7.546355166404728e-06, 3.7823374586042584e-06, -4.4403751281050637e-07, -4.751935226668256e-06, -8.657610605437433e-06, -1.1704235245796244e-05, -1.3598371925425724e-05, -1.4317719739827113e-05, -1.4028976959417443e-05, -1.2833958499471945e-05, -1.0675853285235335e-05, -7.799257503603087e-06, -4.4152270022027145e-06, -6.574369510428113e-07, 3.066186213394877e-06, 6.518108735080605e-06, 9.499645886390903e-06, 1.2004866217787739e-05, 1.4058177002710657e-05, 1.57825580944226e-05, 1.7094462230840832e-05, 1.816168841144271e-05, 1.9149620391624475e-05, 1.987759486932103e-05, 2.0575136550998138e-05, 2.1086597517771753e-05, 2.1538050875364152e-05, 2.1895834079631733e-05, 2.2090003826420656e-05, 2.2472777102214437e-05, 2.2748185039994777e-05, 2.3149346051004747e-05, 2.3503157281721394e-05, 2.188230624454934e-05, 2.2090003826420656e-05], [0.0007561535308541753, 0.0007571495388107443, 0.0007580898249034037, 0.0007589806138682876, 0.0007598273093316671, 0.000760634629787791, 0.0007614827265553315, 0.00076239082489488, 0.0007633208250386864, 0.0007642708121285032, 0.0007653910718702335, 0.0007665011295030483, 0.0007675897166617615, 0.0007687607635486495, 0.0007697944818268928, 0.0007704390632326482, 0.0007704572531665726, 0.0007696971764294077, 0.0007677668668633878, 0.0007646106351609047, 0.0007604223886194601, 0.0007555096365670425, 0.0007504261129548216, 0.0007453854317004968, 0.0007407051018979533, 0.0007364298636975408, 0.0007328800480898012, 0.0007300274269232681, 0.000728148050542536, 0.0007271956502786209, 0.0007270539001216064, 0.0007275615945585623, 0.0007283277849731791, 0.0007292584045472654, 0.0007301880899271334, 0.0007311923243044495, 0.0007321523599595834, 0.0007330968637747902, 0.0007339411268379382, 0.0007347914330913237, 0.0007354838134440733, 0.0007362471882012419, 0.0007369000346289303, 0.0007373279625784092, 0.0007380527615755541, 0.0007386072142055366, 0.0007394320987804113, 0.0007401536167788356, 0.0007368482576083138, 0.0007373279625784092]}, {[2.450174023832185e-05, 2.4452996808547243e-05, 2.4306958887271984e-05, 2.406420281945297e-05, 2.372568665238518e-05, 2.329274635472671e-05, 2.2767090544040805e-05, 2.215079374366295e-05, 2.144628819550501e-05, 2.0656354261107594e-05, 1.9784109448823284e-05, 1.883299611043541e-05, 1.7806767855768246e-05, 1.6709474738903864e-05, 1.554544727446899e-05, 1.4319279347072183e-05, 1.3035810081340042e-05, 1.1700104744103075e-05, 1.0317434754101639e-05, 8.89325687810443e-06, 7.4331916955430365e-06, 5.943001416652686e-06, 4.428567141660986e-06, 2.895865650772125e-06, 1.3509458165459259e-06, -2.0009526823864977e-07, -1.7511363530232198e-06, -3.296056187249419e-06, -4.828757678138285e-06, -6.34319195312998e-06, -7.83338223202033e-06, -9.293447414581725e-06, -1.0717625290578932e-05, -1.2100295280580373e-05, -1.3436000617817343e-05, -1.4719469883549475e-05, -1.5945637810946284e-05, -1.710966527538116e-05, -1.820695839224554e-05, -1.9233186646912705e-05, -2.0184299985300572e-05, -2.1056544797584886e-05, -2.1846478731982303e-05, -2.2550984280140244e-05, -2.31672810805181e-05, -2.3692936891204e-05, -2.412587718886247e-05, -2.446439335593026e-05, -2.4707149423749276e-05, -2.4853187345024535e-05, -2.490193077479914e-05, -2.4853187345024535e-05, -2.4707149423749276e-05, -2.4464393355930258e-05, -2.412587718886247e-05, -2.3692936891204e-05, -2.3167281080518094e-05, -2.255098428014024e-05, -2.18464787319823e-05, -2.1056544797584883e-05, -2.018429998530057e-05, -1.92331866469127e-05, -1.8206958392245537e-05, -1.7109665275381156e-05, -1.5945637810946277e-05, -1.471946988354948e-05, -1.3436000617817329e-05, -1.210029528058037e-05, -1.0717625290578919e-05, -9.29344741458172e-06, -7.83338223202033e-06, -6.34319195312997e-06, -4.82875767813828e-06, -3.2960561872494034e-06, -1.751136353023215e-06, -2.0009526823865033e-07, 1.350945816545936e-06, 2.895865650772124e-06, 4.428567141661001e-06, 5.943001416652691e-06, 7.43319169554303e-06, 8.89325687810444e-06, 1.0317434754101639e-05, 1.1700104744103088e-05, 1.3035810081340048e-05, 1.43192793470722e-05, 1.5545447274468996e-05, 1.6709474738903864e-05, 1.7806767855768256e-05, 1.8832996110435413e-05, 1.978410944882329e-05, 2.06563542611076e-05, 2.144628819550501e-05, 2.2150793743662956e-05, 2.276709054404081e-05, 2.3292746354726713e-05, 2.3725686652385183e-05, 2.406420281945297e-05, 2.4306958887271984e-05, 2.4452996808547243e-05], [0.000748870641466097, 0.0007504216825508816, 0.0007519666023851078, 0.0007534993038759967, 0.0007550137381509884, 0.0007565039284298787, 0.0007579639936124401, 0.0007593881714884373, 0.0007607708414784388, 0.0007621065468156758, 0.0007633900160814079, 0.0007646161840088047, 0.0007657802114732395, 0.000766877504590104, 0.0007679037328447711, 0.0007688548461831589, 0.0007697270909954433, 0.0007705170249298407, 0.0007712215304779987, 0.0007718378272783765, 0.0007723634830890624, 0.0007727964233867208, 0.0007731349395537887, 0.0007733776956216076, 0.0007735237335428829, 0.0007735724769726575, 0.0007735237335428829, 0.0007733776956216076, 0.0007731349395537887, 0.0007727964233867208, 0.0007723634830890624, 0.0007718378272783765, 0.0007712215304779987, 0.0007705170249298407, 0.0007697270909954433, 0.0007688548461831589, 0.0007679037328447711, 0.000766877504590104, 0.0007657802114732395, 0.0007646161840088047, 0.0007633900160814079, 0.0007621065468156758, 0.0007607708414784388, 0.0007593881714884373, 0.0007579639936124401, 0.0007565039284298787, 0.0007550137381509884, 0.0007534993038759967, 0.0007519666023851078, 0.0007504216825508816, 0.000748870641466097, 0.0007473196003813125, 0.0007457746805470863, 0.0007442419790561974, 0.0007427275447812057, 0.0007412373545023154, 0.000739777289319754, 0.0007383531114437568, 0.0007369704414537553, 0.0007356347361165183, 0.0007343512668507862, 0.0007331250989233894, 0.0007319610714589546, 0.0007308637783420901, 0.000729837550087423, 0.0007288864367490351, 0.0007280141919367508, 0.0007272242580023534, 0.0007265197524541954, 0.0007259034556538176, 0.0007253777998431316, 0.0007249448595454733, 0.0007246063433784054, 0.0007243635873105865, 0.0007242175493893112, 0.0007241688059595366, 0.0007242175493893112, 0.0007243635873105865, 0.0007246063433784054, 0.0007249448595454733, 0.0007253777998431316, 0.0007259034556538176, 0.0007265197524541954, 0.0007272242580023534, 0.0007280141919367508, 0.0007288864367490351, 0.000729837550087423, 0.0007308637783420901, 0.0007319610714589546, 0.0007331250989233894, 0.0007343512668507862, 0.0007356347361165183, 0.0007369704414537553, 0.0007383531114437568, 0.000739777289319754, 0.0007412373545023154, 0.0007427275447812057, 0.0007442419790561974, 0.0007457746805470863, 0.0007473196003813125]}, {[8.774239668133993e-06, -1.1892913069245972e-05, 1.2065956309458103e-05], [-1.3749692793169803e-05, 1.2199146161525655e-06, -6.7277510001537665e-06]}, {[9.039245085089989e-06, 9.186842716839702e-06, 9.334440348589416e-06, 9.48203798033913e-06, 9.629635612088843e-06, 9.777233243838556e-06, 9.92483087558827e-06, 1.0072428507337984e-05, 1.0220026139087697e-05, 1.036762377083741e-05, 1.0515221402587124e-05, 1.066281903433684e-05, 1.0810416666086551e-05, 1.0958014297836267e-05, 1.110561192958598e-05, 1.1253209561335694e-05, 1.1400807193085408e-05, 1.1548404824835121e-05, 1.1696002456584835e-05, 1.1843600088334548e-05], [-1.3129000016103014e-05, -1.2830263439856925e-05, -1.2531526863610837e-05, -1.2232790287364749e-05, -1.193405371111866e-05, -1.1635317134872572e-05, -1.1336580558626483e-05, -1.1037843982380395e-05, -1.0739107406134307e-05, -1.0440370829888218e-05, -1.014163425364213e-05, -9.84289767739604e-06, -9.544161101149951e-06, -9.245424524903863e-06, -8.946687948657775e-06, -8.647951372411686e-06, -8.349214796165598e-06, -8.05047821991951e-06, -7.751741643673421e-06, -7.453005067427333e-06]}, {[-1.1892913069245972e-05, -1.1549693415800066e-05, -1.1206473762354162e-05, -1.0863254108908256e-05, -1.0520034455462352e-05, -1.0176814802016447e-05, -9.833595148570543e-06, -9.490375495124637e-06, -9.147155841678733e-06, -8.803936188232827e-06, -8.460716534786923e-06, -8.117496881341018e-06, -7.774277227895114e-06, -7.431057574449208e-06, -7.087837921003303e-06, -6.7446182675573986e-06, -6.401398614111494e-06, -6.058178960665589e-06, -5.714959307219684e-06, -5.371739653773779e-06], [1.2199146161525655e-06, 1.2199146161525655e-06, 1.2199146161525655e-06, 1.2199146161525655e-06, 1.2199146161525655e-06, 1.2199146161525655e-06, 1.2199146161525655e-06, 1.2199146161525655e-06, 1.2199146161525655e-06, 1.2199146161525655e-06, 1.2199146161525655e-06, 1.2199146161525655e-06, 1.2199146161525655e-06, 1.2199146161525655e-06, 1.2199146161525655e-06, 1.2199146161525655e-06, 1.2199146161525655e-06, 1.2199146161525655e-06, 1.2199146161525655e-06, 1.2199146161525655e-06]}]
  out "Plot: dz/domega":cluster{"omega out":dbl[], dbl[]}(graph)={"omega out"=[1993203.2327275807, 1993284.831541473, 1993361.8652934371, 1993434.843950368, 1993504.210209025, 1993570.3506361335, 1993633.604695191, 1993694.2721197682, 1993752.6189752219, 1993808.8826808098, 1993863.276194716, 1993915.991524844, 1993967.2026947618, 1994017.0682615843, 1994065.733471473, 1994113.3321128746, 1994159.9881239824, 1994205.8169966259, 1994250.9270102703, 1994295.4203281004, 1994339.393978848, 1994382.940745254, 1994426.14997686, 1994469.108344603, 1994511.9005478774, 1994554.6099904731, 1994597.3194328558, 1994640.1116363432, 1994683.0700038732, 1994726.2792356922, 1994769.8260018853, 1994813.7996526328, 1994858.2929704627, 1994903.4029841074, 1994949.2318567508, 1994995.887868072, 1995043.4865092603, 1995092.151719149, 1995142.0172861845, 1995193.2284558893, 1995245.9437862302, 1995300.3372999234, 1995356.6010057244, 1995414.9478611783, 1995475.6152855423, 1995538.8693448128, 1995605.0097717082, 1995674.3760305785, 1995747.354687296, 1995824.3884394732], [0.0005491886745889432, 0.0005491886745889432, 0.0005491886745889432, 0.0005491886745889432, 0.0005491886745889432, 0.0005491886745889432, 0.0006115983935948684, 0.0006716930261965111, 0.0007592898100878731, 0.000889528482423159, 0.0010341729357213041, 0.0012461142691368565, 0.0014964746004273582, 0.0018026087445251141, 0.0021619347204561434, 0.0026207202642377866, 0.0031278480421146502, 0.0036845382729539257, 0.004267864752409711, 0.004807398153059608, 0.005260603930209542, 0.005643213616022912, 0.005907516513943102, 0.005989911841595364, 0.005902056007102832, 0.005719709733522932, 0.005395222407433278, 0.0048955426360843945, 0.004331359617424871, 0.003750063808537518, 0.0032072930412866897, 0.0027360980290858936, 0.002338184222132599, 0.0019713487669855614, 0.0016423363464027957, 0.0013840908048551237, 0.0011724647490556123, 0.0010002810323922922, 0.0008609635217160542, 0.000777408284325375, 0.0006736756349363545, 0.0006384825796425174, 0.0005625298517843271, 0.00047076885600725964, 0.0004052750696957624, 0.00044188584837624354, 0.0004689879020460978, 0.0004689879020460978, 0.0004689879020460978, 0.00047076885600725964]}
  out "Plot: win omega":T5(graph)={"omega out"=[1993203.2327275807, 1993284.831541473, 1993361.8652934371, 1993434.843950368, 1993504.210209025, 1993570.3506361335, 1993633.604695191, 1993694.2721197682, 1993752.6189752219, 1993808.8826808098, 1993863.276194716, 1993915.991524844, 1993967.2026947618, 1994017.0682615843, 1994065.733471473, 1994113.3321128746, 1994159.9881239824, 1994205.8169966259, 1994250.9270102703, 1994295.4203281004, 1994339.393978848, 1994382.940745254, 1994426.14997686, 1994469.108344603, 1994511.9005478774, 1994554.6099904731, 1994597.3194328558, 1994640.1116363432, 1994683.0700038732, 1994726.2792356922, 1994769.8260018853, 1994813.7996526328, 1994858.2929704627, 1994903.4029841074, 1994949.2318567508, 1994995.887868072, 1995043.4865092603, 1995092.151719149, 1995142.0172861845, 1995193.2284558893, 1995245.9437862302, 1995300.3372999234, 1995356.6010057244, 1995414.9478611783, 1995475.6152855423, 1995538.8693448128, 1995605.0097717082, 1995674.3760305785, 1995747.354687296, 1995824.3884394732], "win omega out"=[660.0434671354014, 660.0434671354014, 660.0434671354014, 660.0434671354014, 660.0434671354014, 660.0434671354014, 631.1599833709188, 605.3374013246503, 582.2243112162687, 561.5232624479104, 542.9814767411444, 526.3834287915379, 511.5448768576607, 498.30803504842333, 486.53764729062095, 476.117784131784, 466.9492204100825, 458.9472820982337, 452.04008301883005, 446.1670764044393, 441.27787759853527, 437.3313088733703, 434.29463971732184, 432.1429936029017, 430.8589075917844, 430.43202303745784, 430.85890737874433, 432.14299360266887, 434.2946395042818, 437.3313088733703, 441.2778775987681, 446.1670764044393, 452.04008280579, 458.94728231127374, 466.94922019704245, 476.11778434482403, 486.53764729062095, 498.3080352616962, 511.5448770709336, 526.3834287915379, 542.9814767409116, 561.5232624479104, 582.2243114295416, 605.3374011116102, 682.3711532887537, 732.2367203242611, 732.2367203242611, 732.2367203242611, 732.2367203242611, 682.3711532887537]}
  out "Plot: phase":cluster{"omega out":dbl[], dbl[]}(graph)={"omega out"=[1993203.2327275807, 1993284.831541473, 1993361.8652934371, 1993434.843950368, 1993504.210209025, 1993570.3506361335, 1993633.604695191, 1993694.2721197682, 1993752.6189752219, 1993808.8826808098, 1993863.276194716, 1993915.991524844, 1993967.2026947618, 1994017.0682615843, 1994065.733471473, 1994113.3321128746, 1994159.9881239824, 1994205.8169966259, 1994250.9270102703, 1994295.4203281004, 1994339.393978848, 1994382.940745254, 1994426.14997686, 1994469.108344603, 1994511.9005478774, 1994554.6099904731, 1994597.3194328558, 1994640.1116363432, 1994683.0700038732, 1994726.2792356922, 1994769.8260018853, 1994813.7996526328, 1994858.2929704627, 1994903.4029841074, 1994949.2318567508, 1994995.887868072, 1995043.4865092603, 1995092.151719149, 1995142.0172861845, 1995193.2284558893, 1995245.9437862302, 1995300.3372999234, 1995356.6010057244, 1995414.9478611783, 1995475.6152855423, 1995538.8693448128, 1995605.0097717082, 1995674.3760305785, 1995747.354687296, 1995824.3884394732], [-2.8808933940451578, -2.814217663665282, -2.751610919134133, -2.6930480962627037, -2.638411048298231, -2.5875172250982, -2.5335470983278134, -2.4756088418342417, -2.4124056673207224, -2.3448475069135695, -2.2624443225006985, -2.1728467531557265, -2.0701544635204545, -1.9536184015208578, -1.8204045437238803, -1.671491664378478, -1.4985215784774712, -1.3067808805264511, -1.1003244637506706, -0.8838758422741286, -0.6623523644211966, -0.437298269078342, -0.21705037966130147, 0.0, 0.20709623120173148, 0.41180773412047955, 0.606989009318696, 0.796152587471771, 0.9763391355989994, 1.1427442621376986, 1.294217231988262, 1.4285801395313271, 1.5481373158803047, 1.6532348472942813, 1.7471773924961989, 1.8266498868941996, 1.8970728155297412, 1.9660580078638965, 2.0227411434718157, 2.079966830811233, 2.1253153227220016, 2.1719097579178026, 2.2116444636676356, 2.2366376529940073, 2.2818550407093987, 2.3164335004111534, 2.368466461257648, 2.4147752096594335, 2.209034538666793, 2.2366376529940073]}
  out "Plot: phase around center":cluster{dbl[], dbl[]}[](graph)=[{[1993203.2327275807, 1993284.831541473, 1993361.8652934371, 1993434.843950368, 1993504.210209025, 1993570.3506361335, 1993633.604695191, 1993694.2721197682, 1993752.6189752219, 1993808.8826808098, 1993863.276194716, 1993915.991524844, 1993967.2026947618, 1994017.0682615843, 1994065.733471473, 1994113.3321128746, 1994159.9881239824, 1994205.8169966259, 1994250.9270102703, 1994295.4203281004, 1994339.393978848, 1994382.940745254, 1994426.14997686, 1994469.108344603, 1994511.9005478774, 1994554.6099904731, 1994597.3194328558, 1994640.1116363432, 1994683.0700038732, 1994726.2792356922, 1994769.8260018853, 1994813.7996526328, 1994858.2929704627, 1994903.4029841074, 1994949.2318567508, 1994995.887868072, 1995043.4865092603, 1995092.151719149, 1995142.0172861845, 1995193.2284558893, 1995245.9437862302, 1995300.3372999234, 1995356.6010057244, 1995414.9478611783, 1995475.6152855423, 1995538.8693448128, 1995605.0097717082, 1995674.3760305785, 1995747.354687296, 1995824.3884394732], [-2.561448603269745, -2.522526300435735, -2.48085148055218, -2.4360720803752978, -2.3877811643485134, -2.3355072109282156, -2.2787028465281196, -2.216732014277936, -2.148855798648791, -2.0742175451169125, -1.991828681830962, -1.9005579324952873, -1.7991286826393664, -1.6861324230085561, -1.5600705422045038, -1.4194418888157165, -1.2628974808525855, -1.0894818519964762, -0.8989643994906764, -0.6922242107374568, -0.4715880284978294, -0.24096027814647478, -0.005586951393884288, 0.2285851533612811, 0.45579058173655806, 0.6712630493757283, 0.8717225137419554, 1.0554510983761682, 1.2220586990410163, 1.3721097623376366, 1.5067517186161565, 1.6274180201908046, 1.7356230992605721, 1.8328371074387684, 1.9204190212377297, 1.9995879567851655, 2.071417342455842, 2.1368415533028444, 2.196668484171495, 2.251594244384857, 2.302217874090718, 2.3490550293008523, 2.392550200333962, 2.433087347707029, 2.47099902647123, 2.506574137229946, 2.5400644754300026, 2.5716902506741186, 2.601644729881701, 2.6300981476334733]}, {[1993203.2327275807, 1993284.831541473, 1993361.8652934371, 1993434.843950368, 1993504.210209025, 1993570.3506361335, 1993633.604695191, 1993694.2721197682, 1993752.6189752219, 1993808.8826808098, 1993863.276194716, 1993915.991524844, 1993967.2026947618, 1994017.0682615843, 1994065.733471473, 1994113.3321128746, 1994159.9881239824, 1994205.8169966259, 1994250.9270102703, 1994295.4203281004, 1994339.393978848, 1994382.940745254, 1994426.14997686, 1994469.108344603, 1994511.9005478774, 1994554.6099904731, 1994597.3194328558, 1994640.1116363432, 1994683.0700038732, 1994726.2792356922, 1994769.8260018853, 1994813.7996526328, 1994858.2929704627, 1994903.4029841074, 1994949.2318567508, 1994995.887868072, 1995043.4865092603, 1995092.151719149, 1995142.0172861845, 1995193.2284558893, 1995245.9437862302, 1995300.3372999234, 1995356.6010057244, 1995414.9478611783, 1995475.6152855423, 1995538.8693448128, 1995605.0097717082, 1995674.3760305785, 1995747.354687296, 1995824.3884394732], [-2.8808933940451578, -2.814217663665282, -2.751610919134133, -2.6930480962627037, -2.638411048298231, -2.5875172250982, -2.5335470983278134, -2.4756088418342417, -2.4124056673207224, -2.3448475069135695, -2.2624443225006985, -2.1728467531557265, -2.0701544635204545, -1.9536184015208578, -1.8204045437238803, -1.671491664378478, -1.4985215784774712, -1.3067808805264511, -1.1003244637506706, -0.8838758422741286, -0.6623523644211966, -0.437298269078342, -0.21705037966130147, 0.0, 0.20709623120173148, 0.41180773412047955, 0.606989009318696, 0.796152587471771, 0.9763391355989994, 1.1427442621376986, 1.294217231988262, 1.4285801395313271, 1.5481373158803047, 1.6532348472942813, 1.7471773924961989, 1.8266498868941996, 1.8970728155297412, 1.9660580078638965, 2.0227411434718157, 2.079966830811233, 2.1253153227220016, 2.1719097579178026, 2.2116444636676356, 2.2366376529940073, 2.2818550407093987, 2.3164335004111534, 2.368466461257648, 2.4147752096594335, 2.209034538666793, 2.2366376529940073]}]
  out "Plot: fragment":cluster{dbl[], dbl[]}[](graph)=[{[1993203.2327275807, 1993284.831541473, 1993361.8652934371, 1993434.843950368, 1993504.210209025, 1993570.3506361335, 1993633.604695191, 1993694.2721197682, 1993752.6189752219, 1993808.8826808098, 1993863.276194716, 1993915.991524844, 1993967.2026947618, 1994017.0682615843, 1994065.733471473, 1994113.3321128746, 1994159.9881239824, 1994205.8169966259, 1994250.9270102703, 1994295.4203281004, 1994339.393978848, 1994382.940745254, 1994426.14997686, 1994469.108344603, 1994511.9005478774, 1994554.6099904731, 1994597.3194328558, 1994640.1116363432, 1994683.0700038732, 1994726.2792356922, 1994769.8260018853, 1994813.7996526328, 1994858.2929704627, 1994903.4029841074, 1994949.2318567508, 1994995.887868072, 1995043.4865092603, 1995092.151719149, 1995142.0172861845, 1995193.2284558893, 1995245.9437862302, 1995300.3372999234, 1995356.6010057244, 1995414.9478611783, 1995475.6152855423, 1995538.8693448128, 1995605.0097717082, 1995674.3760305785, 1995747.354687296, 1995824.3884394732], [1.2015131430941288e-05, 1.1934665415056156e-05, 1.1384660360389812e-05, 1.0853505704743488e-05, 1.1153663067501817e-05, 1.015355315583528e-05, 1.018895996788804e-05, 9.703331423021854e-06, 9.144693658415838e-06, 8.09313274780445e-06, 7.677593316262773e-06, 6.794847591763187e-06, 5.14654084207493e-06, 3.5994652431912764e-06, 1.2732245129806887e-06, -1.478733385405568e-06, -4.873358583976242e-06, -8.708631835863113e-06, -1.3972126929153133e-05, -1.9783040901589133e-05, -2.6539857664253126e-05, -3.2353170572386246e-05, -3.5851782447950046e-05, -3.564472919284043e-05, -3.214223119648663e-05, -2.6210211818249885e-05, -1.9913445090203948e-05, -1.4594458434140163e-05, -1.0315819169974256e-05, -5.416042203770771e-06, -2.457205171384409e-06, -2.928970730186009e-07, 2.3172206962110824e-06, 3.886508066355551e-06, 5.366133798595151e-06, 6.49061925361229e-06, 7.565434276920878e-06, 8.07146540316344e-06, 8.774239668133993e-06, 9.031647316981642e-06, 9.336145185069177e-06, 1.0413063973015958e-05, 1.0259874367567215e-05, 1.1251324735561457e-05, 1.0901407495319138e-05, 1.1298829983199349e-05, 1.1368515397924067e-05, 1.1202845721581676e-05, 1.1829541584104692e-05, 1.2065956309458103e-05]}, {[1993203.2327275807, 1993284.831541473, 1993361.8652934371, 1993434.843950368, 1993504.210209025, 1993570.3506361335, 1993633.604695191, 1993694.2721197682, 1993752.6189752219, 1993808.8826808098, 1993863.276194716, 1993915.991524844, 1993967.2026947618, 1994017.0682615843, 1994065.733471473, 1994113.3321128746, 1994159.9881239824, 1994205.8169966259, 1994250.9270102703, 1994295.4203281004, 1994339.393978848, 1994382.940745254, 1994426.14997686, 1994469.108344603, 1994511.9005478774, 1994554.6099904731, 1994597.3194328558, 1994640.1116363432, 1994683.0700038732, 1994726.2792356922, 1994769.8260018853, 1994813.7996526328, 1994858.2929704627, 1994903.4029841074, 1994949.2318567508, 1994995.887868072, 1995043.4865092603, 1995092.151719149, 1995142.0172861845, 1995193.2284558893, 1995245.9437862302, 1995300.3372999234, 1995356.6010057244, 1995414.9478611783, 1995475.6152855423, 1995538.8693448128, 1995605.0097717082, 1995674.3760305785, 1995747.354687296, 1995824.3884394732], [9.021960124832402e-06, 9.490365587486302e-06, 1.0321922687315643e-05, 1.1438913182656562e-05, 1.1545749602055082e-05, 1.2703793323099355e-05, 1.3738928411510115e-05, 1.4340634913292461e-05, 1.4879304206685535e-05, 1.6806176108942494e-05, 1.7322609182562855e-05, 1.845529204474582e-05, 1.9486013878596822e-05, 2.063086375145935e-05, 2.2492750316338074e-05, 2.353379538528439e-05, 2.4431588274432528e-05, 2.5921750122713007e-05, 2.575641497357074e-05, 2.4248100999623746e-05, 2.008380027019457e-05, 1.4763861911080045e-05, 6.0099803757352e-06, -3.66978837051642e-06, -1.2092065197376258e-05, -1.906240691515503e-05, -2.2184322081616873e-05, -2.3481920890407984e-05, -2.3185624603622515e-05, -2.3109632069119373e-05, -2.1739456958141576e-05, -2.0872603959020937e-05, -1.9341414526159468e-05, -1.8227183731143147e-05, -1.6919143618833086e-05, -1.5728397329680018e-05, -1.521527017191973e-05, -1.4309611421280035e-05, -1.3749692793169803e-05, -1.2714231525831209e-05, -1.1847546684768469e-05, -1.1068060741260257e-05, -1.0584091713681035e-05, -9.522992305577424e-06, -9.685277353777368e-06, -8.089635084054e-06, -8.399762072942157e-06, -8.401069770179004e-06, -7.495616744822688e-06, -6.7277510001537665e-06]}, {[1993203.2327275807, 1993284.831541473, 1993361.8652934371, 1993434.843950368, 1993504.210209025, 1993570.3506361335, 1993633.604695191, 1993694.2721197682, 1993752.6189752219, 1993808.8826808098, 1993863.276194716, 1993915.991524844, 1993967.2026947618, 1994017.0682615843, 1994065.733471473, 1994113.3321128746, 1994159.9881239824, 1994205.8169966259, 1994250.9270102703, 1994295.4203281004, 1994339.393978848, 1994382.940745254, 1994426.14997686, 1994469.108344603, 1994511.9005478774, 1994554.6099904731, 1994597.3194328558, 1994640.1116363432, 1994683.0700038732, 1994726.2792356922, 1994769.8260018853, 1994813.7996526328, 1994858.2929704627, 1994903.4029841074, 1994949.2318567508, 1994995.887868072, 1995043.4865092603, 1995092.151719149, 1995142.0172861845, 1995193.2284558893, 1995245.9437862302, 1995300.3372999234, 1995356.6010057244, 1995414.9478611783, 1995475.6152855423, 1995538.8693448128, 1995605.0097717082, 1995674.3760305785, 1995747.354687296, 1995824.3884394732], [1.388596045541361e-05, 1.344602210924949e-05, 1.2944699332950554e-05, 1.2372113651060794e-05, 1.1716544711752725e-05, 1.0964094065618954e-05, 1.0098316412632153e-05, 9.099842572493444e-06, 7.946046305651416e-06, 6.610855216710278e-06, 5.06488663739989e-06, 3.2762175533780364e-06, 1.2122885191787847e-06, -1.1563037830444422e-06, -3.8491016249455735e-06, -6.865031105874085e-06, -1.0166903296989207e-05, -1.3662184307126868e-05, -1.7184779195562985e-05, -2.0488095286775392e-05, -2.326373292858256e-05, -2.519577135444693e-05, -2.6042228762580408e-05, -2.571056032107456e-05, -2.4286321610940307e-05, -2.19986387380212e-05, -1.9144725269827595e-05, -1.6013907976187713e-05, -1.2839356362871063e-05, -9.782172466272873e-06, -6.937599187245625e-06, -4.350688732291268e-06, -2.032818841950683e-06, 2.4852587767243742e-08, 1.8418515965701254e-06, 3.4422437146042875e-06, 4.850978652054634e-06, 6.091894702625287e-06, 7.186757352147025e-06, 8.15490662160849e-06, 9.013241459427858e-06, 9.776375756714944e-06, 1.0456869515886518e-05, 1.1065481081348542e-05, 1.161141215858856e-05, 1.2102532031320777e-05, 1.2545575855256362e-05, 1.2946316400102913e-05, 1.3309710799253384e-05, 1.3640024950759725e-05]}, {[1993203.2327275807, 1993284.831541473, 1993361.8652934371, 1993434.843950368, 1993504.210209025, 1993570.3506361335, 1993633.604695191, 1993694.2721197682, 1993752.6189752219, 1993808.8826808098, 1993863.276194716, 1993915.991524844, 1993967.2026947618, 1994017.0682615843, 1994065.733471473, 1994113.3321128746, 1994159.9881239824, 1994205.8169966259, 1994250.9270102703, 1994295.4203281004, 1994339.393978848, 1994382.940745254, 1994426.14997686, 1994469.108344603, 1994511.9005478774, 1994554.6099904731, 1994597.3194328558, 1994640.1116363432, 1994683.0700038732, 1994726.2792356922, 1994769.8260018853, 1994813.7996526328, 1994858.2929704627, 1994903.4029841074, 1994949.2318567508, 1994995.887868072, 1995043.4865092603, 1995092.151719149, 1995142.0172861845, 1995193.2284558893, 1995245.9437862302, 1995300.3372999234, 1995356.6010057244, 1995414.9478611783, 1995475.6152855423, 1995538.8693448128, 1995605.0097717082, 1995674.3760305785, 1995747.354687296, 1995824.3884394732], [1.2533111386283128e-05, 1.3243870686753404e-05, 1.398529142825186e-05, 1.4757913883288497e-05, 1.5561486507967032e-05, 1.6394557133308867e-05, 1.7253890955446958e-05, 1.8133647726468528e-05, 1.9024228688692738e-05, 1.9910680787311335e-05, 2.0770528532712855e-05, 2.157091107424648e-05, 2.22649712916139e-05, 2.2787646339351097e-05, 2.3051462385800282e-05, 2.2943790381521937e-05, 2.23283645267604e-05, 2.105544743308328e-05, 1.8985726685443274e-05, 1.60304361745741e-05, 1.2201584487660623e-05, 7.65254974905696e-06, 2.680539472875356e-06, -2.3264138334989134e-06, -6.982761496284861e-06, -1.0995269066542239e-05, -1.4209180601135879e-05, -1.6601931437915606e-05, -1.8244142944012906e-05, -1.9254094178099146e-05, -1.976208567613664e-05, -1.988911600601874e-05, -1.973738050044325e-05, -1.938823379296975e-05, -1.8903943642141984e-05, -1.833087853442706e-05, -1.7702870514378437e-05, -1.704419860290617e-05, -1.6372021597483308e-05, -1.569826943722966e-05, -1.503107177976094e-05, -1.4375817771313947e-05, -1.3735933215610978e-05, -1.3113446439454667e-05, -1.2509398299166067e-05, -1.1924138345739232e-05, -1.1357538215222098e-05, -1.0809144984910333e-05, -1.027829111604876e-05, -9.764172916798281e-06]}]
  out "Plot: complex plane":cluster{dbl[], dbl[]}[](graph)=[{[2.3707949231948613e-05, 2.3627483216063482e-05, 2.3077478161397138e-05, 2.2546323505750814e-05, 2.2846480868509143e-05, 2.1846370956842606e-05, 2.1881777768895366e-05, 2.139614922402918e-05, 2.0837511459423164e-05, 1.9785950548811776e-05, 1.93704111172701e-05, 1.8487665392770513e-05, 1.6839358643082255e-05, 1.5292283044198602e-05, 1.2966042313988014e-05, 1.0214084415601758e-05, 6.819459217031084e-06, 2.9841859651442124e-06, -2.279309128145807e-06, -8.090223100581807e-06, -1.48470398632458e-05, -2.066035277137892e-05, -2.415896464694272e-05, -2.39519113918331e-05, -2.0449413395479304e-05, -1.451739401724256e-05, -8.220627289196623e-06, -2.9016406331328374e-06, 1.3769986310330693e-06, 6.276775597236554e-06, 9.235612629622917e-06, 1.1399920727988725e-05, 1.4010038497218408e-05, 1.5579325867362877e-05, 1.7058951599602477e-05, 1.8183437054619616e-05, 1.9258252077928204e-05, 1.9764283204170766e-05, 2.046705746914132e-05, 2.0724465117988968e-05, 2.1028962986076503e-05, 2.2105881774023284e-05, 2.195269216857454e-05, 2.2944142536568783e-05, 2.2594225296326463e-05, 2.2991647784206674e-05, 2.3061333198931392e-05, 2.2895663522589002e-05, 2.3522359385112018e-05, 2.3758774110465428e-05], [0.0007566726869747769, 0.0007571410924374308, 0.0007579726495372601, 0.000759089640032601, 0.0007591964764519996, 0.0007603545201730438, 0.0007613896552614546, 0.0007619913617632369, 0.00076253003105663, 0.000764456902958887, 0.0007649733360325073, 0.0007661060188946903, 0.0007671367407285413, 0.0007682815906014038, 0.0007701434771662825, 0.0007711845222352289, 0.000772082315124377, 0.0007735724769726575, 0.0007734071418235152, 0.0007718988278495682, 0.000767734527120139, 0.0007624145887610245, 0.0007536607072256797, 0.0007439809384794281, 0.0007355586616525682, 0.0007285883199347894, 0.0007254664047683276, 0.0007241688059595365, 0.000724465102246322, 0.0007245410947808251, 0.0007259112698918029, 0.0007267781228909235, 0.000728309312323785, 0.0007294235431188013, 0.0007307315832311114, 0.0007319223295202645, 0.0007324354566780247, 0.0007333411154286644, 0.0007339010340567747, 0.0007349364953241133, 0.000735803180165176, 0.0007365826661086842, 0.0007370666351362634, 0.000738127734544367, 0.0007379654494961671, 0.0007395610917658905, 0.0007392509647770023, 0.0007392496570797655, 0.0007401551101051218, 0.0007409229758497907]}, {[2.8577545646642735e-05, 2.8408189863685476e-05, 2.7902793356679178e-05, 2.706932653044857e-05, 2.5920933654732258e-05, 2.4475725571196938e-05, 2.275649407464542e-05, 2.079035247279744e-05, 1.8608307993230206e-05, 1.624477278087668e-05, 1.3737021197943175e-05, 1.112460198495073e-05, 8.448714553471839e-06, 5.751559246798586e-06, 3.0756718153196897e-06, 4.6325260232724873e-07, -2.044498980606255e-06, -4.408034192959786e-06, -6.5900786725270175e-06, -8.556220274374998e-06, -1.0275451770926508e-05, -1.1720659854461832e-05, -1.2869052730178146e-05, -1.3702519556408752e-05, -1.420791606341505e-05, -1.4377271846372308e-05, -1.420791606341505e-05, -1.3702519556408752e-05, -1.2869052730178142e-05, -1.1720659854461828e-05, -1.0275451770926504e-05, -8.556220274374994e-06, -6.590078672527012e-06, -4.408034192959774e-06, -2.0444989806062433e-06, 4.6325260232724873e-07, 3.075671815319694e-06, 5.75155924679859e-06, 8.448714553471847e-06, 1.1124601984950743e-05, 1.373702119794317e-05, 1.624477278087668e-05, 1.8608307993230212e-05, 2.0790352472797446e-05, 2.2756494074645427e-05, 2.4475725571196944e-05, 2.5920933654732258e-05, 2.7069326530448572e-05, 2.790279335667918e-05, 2.8408189863685476e-05], [0.000749237656249328, 0.0007519294893361101, 0.0007545788706070904, 0.0007571440177369621, 0.0007595844768231424, 0.0007618617603679825, 0.0007639399542495972, 0.0007657862841090207, 0.0007673716322214256, 0.0007686709967000383, 0.0007696638857908286, 0.0007703346410397112, 0.0007706726842357217, 0.0007706726842357217, 0.0007703346410397112, 0.0007696638857908286, 0.0007686709967000383, 0.0007673716322214256, 0.0007657862841090207, 0.0007639399542495972, 0.0007618617603679825, 0.0007595844768231424, 0.0007571440177369621, 0.0007545788706070904, 0.0007519294893361101, 0.000749237656249328, 0.000746545823162546, 0.0007438964418915656, 0.0007413312947616939, 0.0007388908356755137, 0.0007366135521306735, 0.0007345353582490588, 0.0007326890283896354, 0.0007311036802772305, 0.0007298043157986177, 0.0007288114267078275, 0.0007281406714589448, 0.0007278026282629343, 0.0007278026282629343, 0.0007281406714589448, 0.0007288114267078275, 0.0007298043157986177, 0.0007311036802772305, 0.0007326890283896354, 0.0007345353582490588, 0.0007366135521306735, 0.0007388908356755137, 0.0007413312947616939, 0.0007438964418915656, 0.000746545823162546]}, {[2.855545991388178e-05, 2.6409927612507122e-05, 2.4264395311132465e-05, 2.211886300975781e-05, 1.9973330708383154e-05, 1.7827798407008496e-05, 1.5682266105633842e-05, 1.3536733804259185e-05, 1.1391201502884528e-05, 9.24566920150987e-06, 7.100136900135213e-06, 4.954604598760559e-06, 2.809072297385902e-06, 6.635399960112447e-07, -1.4819923053634092e-06, -3.6275246067380665e-06, -5.773056908112724e-06, -7.918589209487381e-06, -1.0064121510862038e-05, -1.2209653812236696e-05], [0.000748263900201668, 0.000748361275806434, 0.0007484586514112, 0.000748556027015966, 0.000748653402620732, 0.000748750778225498, 0.000748848153830264, 0.00074894552943503, 0.000749042905039796, 0.000749140280644562, 0.000749237656249328, 0.0007493350318540941, 0.00074943240745886, 0.0007495297830636261, 0.000749627158668392, 0.0007497245342731581, 0.0007498219098779241, 0.00074991928548269, 0.0007500166610874561, 0.000750114036692222]}, {[6.1263808524750964e-06, 6.223756457241108e-06, 6.32113206200712e-06, 6.418507666773131e-06, 6.515883271539143e-06, 6.613258876305155e-06, 6.710634481071167e-06, 6.8080100858371785e-06, 6.9053856906031895e-06, 7.002761295369201e-06, 7.100136900135213e-06, 7.197512504901225e-06, 7.294888109667237e-06, 7.392263714433248e-06, 7.48963931919926e-06, 7.5870149239652715e-06, 7.684390528731283e-06, 7.781766133497294e-06, 7.879141738263306e-06, 7.976517343029318e-06], [0.0007277823332355814, 0.0007299278655369561, 0.0007320733978383307, 0.0007342189301397054, 0.0007363644624410801, 0.0007385099947424547, 0.0007406555270438294, 0.0007428010593452041, 0.0007449465916465788, 0.0007470921239479533, 0.000749237656249328, 0.0007513831885507027, 0.0007535287208520773, 0.000755674253153452, 0.0007578197854548267, 0.0007599653177562014, 0.000762110850057576, 0.0007642563823589506, 0.0007664019146603253, 0.0007685474469616999]}, {[-0.1281782409682419, -0.1293005981432667, -0.13034213934573763, -0.13130221364630673, -0.13218022102978796, -0.13297561277014697, -0.1336878917734372, -0.13431661288846725, -0.13486138318500598, -0.1353218621993511, -0.13569776214710788, -0.13598884810304504, -0.13619493814791542, -0.13631590348214942, -0.1363516685063508, -0.1363022108685436, -0.13616756147814155, -0.1359478044866306, -0.13564307723497707, -0.13525357016779396], [0.04724907219161791, 0.044030126727123024, 0.04078413112403337, 0.03751311402393911, 0.03421911970605172, 0.030904206809595682, 0.027570447047226204, 0.024219923910276202, 0.02085473136664197, 0.017476972552121658, 0.014088758456023486, 0.010692206601866384, 0.007289439723996662, 0.0038825844409480885, 0.0004737699263747608, -0.0029348734216134743, -0.006341215311880256, -0.009743126891625382, -0.013138482076848574, -0.016525158881082528]}, {[-0.14227913368470663, -0.14352495014898417, -0.14468106088372687, -0.1457467433573586, -0.14672133155302275, -0.14760421638482127, -0.14839484607847342, -0.14909272651615676, -0.14969742154531476, -0.15020855325123783, -0.15062580219324787, -0.15094890760433813, -0.15117766755414425, -0.15131193907514398, -0.1513516382520075, -0.15129674027404152, -0.15114727945069523, -0.15090334919011808, -0.15056510194078268, -0.1501327490962094], [0.05236422855274239, 0.04879119908715306, 0.04518814396772355, 0.041557314986618916, 0.03790098129376392, 0.03422142797869772, 0.030520954642467596, 0.026801873960453092, 0.023066510237019097, 0.01931719795290155, 0.015556280306232576, 0.011786107748118193, 0.008009036513682802, 0.004227427149498884, 0.00044364303832249055, -0.003339951077944451, -0.0071209905761405795, -0.01089711242965767, -0.014665956685255412, -0.0184251679379551]}, {[2.4059415521428895e-05, 2.357635867336631e-05, 2.3120326537076183e-05, 2.2688300159348305e-05, 2.2277658819475025e-05, 2.188611408096243e-05, 2.1424606161526664e-05, 2.0884003468308606e-05, 2.0193354223370333e-05, 1.9374046225661016e-05, 1.8285083420554144e-05, 1.696272915357647e-05, 1.5277396401376255e-05, 1.322664151216894e-05, 1.0652214759659831e-05, 7.546355166404728e-06, 3.7823374586042584e-06, -4.4403751281050637e-07, -4.751935226668256e-06, -8.657610605437433e-06, -1.1704235245796244e-05, -1.3598371925425724e-05, -1.4317719739827113e-05, -1.4028976959417443e-05, -1.2833958499471945e-05, -1.0675853285235335e-05, -7.799257503603087e-06, -4.4152270022027145e-06, -6.574369510428113e-07, 3.066186213394877e-06, 6.518108735080605e-06, 9.499645886390903e-06, 1.2004866217787739e-05, 1.4058177002710657e-05, 1.57825580944226e-05, 1.7094462230840832e-05, 1.816168841144271e-05, 1.9149620391624475e-05, 1.987759486932103e-05, 2.0575136550998138e-05, 2.1086597517771753e-05, 2.1538050875364152e-05, 2.1895834079631733e-05, 2.2090003826420656e-05, 2.2472777102214437e-05, 2.2748185039994777e-05, 2.3149346051004747e-05, 2.3503157281721394e-05, 2.188230624454934e-05, 2.2090003826420656e-05], [0.0007561535308541753, 0.0007571495388107443, 0.0007580898249034037, 0.0007589806138682876, 0.0007598273093316671, 0.000760634629787791, 0.0007614827265553315, 0.00076239082489488, 0.0007633208250386864, 0.0007642708121285032, 0.0007653910718702335, 0.0007665011295030483, 0.0007675897166617615, 0.0007687607635486495, 0.0007697944818268928, 0.0007704390632326482, 0.0007704572531665726, 0.0007696971764294077, 0.0007677668668633878, 0.0007646106351609047, 0.0007604223886194601, 0.0007555096365670425, 0.0007504261129548216, 0.0007453854317004968, 0.0007407051018979533, 0.0007364298636975408, 0.0007328800480898012, 0.0007300274269232681, 0.000728148050542536, 0.0007271956502786209, 0.0007270539001216064, 0.0007275615945585623, 0.0007283277849731791, 0.0007292584045472654, 0.0007301880899271334, 0.0007311923243044495, 0.0007321523599595834, 0.0007330968637747902, 0.0007339411268379382, 0.0007347914330913237, 0.0007354838134440733, 0.0007362471882012419, 0.0007369000346289303, 0.0007373279625784092, 0.0007380527615755541, 0.0007386072142055366, 0.0007394320987804113, 0.0007401536167788356, 0.0007368482576083138, 0.0007373279625784092]}]
  in  "scale gauge: Plot: complex plane":dbl(slide)=0.00013000000000000002 min=0.0 max=0.3 step=1e-05 scale=0.0001..1.0 scale format="%#_2g"
  out "window width (kHz)":dbl=76.27809365793496
  out "window center (kHz)":dbl=3399.029286744401
  out "# of points in window":dbl=953.475933538175
  in  "use fast fit?":bool
  out "pm lorentzian":T6={"Amplitude"=0.015694063068390624, "omega(0)"=1994442.711876669, "Gamma"=726.2192575744249, "phase"=4.674130055301799, "Q"=2746.3126726252153, "Norm  Ampl"=nan, "z (inf)"=2.888664009474911e-05+0.0007484535164981425i, "4corners"={"z (-pi/2)"=6.465216046631384e-06+0.0007276852887987989i, "z(inf)"=2.888664009474911e-05+0.0007484535164981425i, "z (pi/2)"=8.118412395405564e-06+0.0007708749405462602i, "z center"=7.291814221018475e-06+0.0007492801146725296i, "z(0)"=-1.4303011652712163e-05+0.0007501067128469166i, "radius"=2.1610640181601427e-05}} {"z (inf)" format="%#9_9f"; "Q" format="%#9_9f"; "phase" format="%#9_9f"; "Gamma" format="%#9_9f"; "omega(0)" format="%#9_9f"}
  in  "plot staff":enum16{"plot", "do not plot", "a"}(ring)
  out "Freq out":dbl[](array[numeric])=[1907168.346185415, 1965249.3711735276, 1976970.6285003964, 1982011.816659579, 1984821.3372776513, 1986615.362944235, 1987862.2368974418, 1988780.6904674931, 1989486.5864630162, 1990047.0317770669, 1990503.5833778584, 1990883.3521453317, 1991204.7790270294, 1991480.8449781418, 1991720.9531195113, 1991932.0825617604, 1992119.5227900057, 1992287.356339517, 1992438.7849751213, 1992576.3555406206, 1992702.1197279515, 1992817.749276128, 1992924.6204638672, 1993023.8770414377, 1993116.4777602106, 1993203.2327275807, 1993284.831541473, 1993361.8652934371, 1993434.843950368, 1993504.210209025, 1993570.3506361335, 1993633.604695191, 1993694.2721197682, 1993752.6189752219, 1993808.8826808098, 1993863.276194716, 1993915.991524844, 1993967.2026947618, 1994017.0682615843, 1994065.733471473, 1994113.3321128746, 1994159.9881239824, 1994205.8169966259, 1994250.9270102703, 1994295.4203281004, 1994339.393978848, 1994382.940745254, 1994426.14997686, 1994469.108344603, 1994511.9005478774, 1994554.6099904731, 1994597.3194328558, 1994640.1116363432, 1994683.0700038732, 1994726.2792356922, 1994769.8260018853, 1994813.7996526328, 1994858.2929704627, 1994903.4029841074, 1994949.2318567508, 1994995.887868072, 1995043.4865092603, 1995092.151719149, 1995142.0172861845, 1995193.2284558893, 1995245.9437862302, 1995300.3372999234, 1995356.6010057244, 1995414.9478611783, 1995475.6152855423, 1995538.8693448128, 1995605.0097717082, 1995674.3760305785, 1995747.354687296, 1995824.3884394732, 1995905.9872531525, 1995992.7422207356, 1996085.3429392956, 1996184.599517079, 1996291.4707048186, 1996407.1002529948, 1996532.8644403256, 1996670.435005825, 1996821.8636414292, 1996989.6971907276, 1997177.137419186, 1997388.266861222, 1997628.3750028044, 1997904.440953917, 1998225.8678354016, 1998605.636603088, 1999062.1882036664, 1999622.63351793, 2000328.5295134531, 2001246.9830832912, 2002493.8570367112, 2004287.882703082, 2007097.4033211542, 2012138.5914805501]
  out "Voltage out":cdb[](array[numeric])=[2.3267514059577948e-05+0.0007497899281750819i, 2.4909528000811873e-05+0.0007493263849847805i, 2.493131520279196e-05+0.0007496174170895291i, 2.4976654073748857e-05+0.0007494851506398698i, 2.5405139290521606e-05+0.0007499570558175639i, 2.4883129570955604e-05+0.000749671639118597i, 2.512681802676727e-05+0.0007497804737566186i, 2.5324670293110625e-05+0.0007503679858101448i, 2.5110327803608353e-05+0.0007502255702464996i, 2.489327033666908e-05+0.0007506115096857297i, 2.472882726006047e-05+0.0007515632145252575i, 2.4998415038301484e-05+0.0007513210836185486i, 2.500505012592314e-05+0.000751689059960851i, 2.5078583497907004e-05+0.0007518588196943513i, 2.4694152114450753e-05+0.0007527186541816263i, 2.5044541628387363e-05+0.0007526931913545811i, 2.4861233245129487e-05+0.0007527422720404769i, 2.488726435100131e-05+0.0007539103456144731i, 2.4957802482118494e-05+0.0007536834592494241i, 2.46934049440733e-05+0.0007546041049378904i, 2.441914511482881e-05+0.0007547662426987134i, 2.382274155491927e-05+0.0007552009676527804i, 2.414210352196834e-05+0.0007555408747181414i, 2.399883643454102e-05+0.0007557323978014151i, 2.350820965974361e-05+0.0007559722204108125i, 2.3707949231948613e-05+0.0007566726869747769i, 2.3627483216063482e-05+0.0007571410924374308i, 2.3077478161397138e-05+0.0007579726495372601i, 2.2546323505750814e-05+0.000759089640032601i, 2.2846480868509143e-05+0.0007591964764519996i, 2.1846370956842606e-05+0.0007603545201730438i, 2.1881777768895366e-05+0.0007613896552614546i, 2.139614922402918e-05+0.0007619913617632369i, 2.0837511459423164e-05+0.00076253003105663i, 1.9785950548811776e-05+0.000764456902958887i, 1.93704111172701e-05+0.0007649733360325073i, 1.8487665392770513e-05+0.0007661060188946903i, 1.6839358643082255e-05+0.0007671367407285413i, 1.5292283044198602e-05+0.0007682815906014038i, 1.2966042313988014e-05+0.0007701434771662825i, 1.0214084415601758e-05+0.0007711845222352289i, 6.819459217031084e-06+0.000772082315124377i, 2.984185965144213e-06+0.0007735724769726575i, -2.279309128145807e-06+0.0007734071418235152i, -8.090223100581805e-06+0.0007718988278495682i, -1.48470398632458e-05+0.000767734527120139i, -2.0660352771378924e-05+0.0007624145887610245i, -2.415896464694272e-05+0.0007536607072256797i, -2.3951911391833105e-05+0.0007439809384794281i, -2.0449413395479307e-05+0.0007355586616525682i, -1.4517394017242558e-05+0.0007285883199347894i, -8.22062728919662e-06+0.0007254664047683276i, -2.901640633132837e-06+0.0007241688059595365i, 1.3769986310330702e-06+0.000724465102246322i, 6.276775597236554e-06+0.0007245410947808251i, 9.235612629622917e-06+0.0007259112698918029i, 1.1399920727988725e-05+0.0007267781228909235i, 1.4010038497218408e-05+0.000728309312323785i, 1.5579325867362877e-05+0.0007294235431188013i, 1.7058951599602477e-05+0.0007307315832311114i, 1.8183437054619616e-05+0.0007319223295202645i, 1.9258252077928204e-05+0.0007324354566780247i, 1.9764283204170766e-05+0.0007333411154286644i, 2.046705746914132e-05+0.0007339010340567747i, 2.0724465117988968e-05+0.0007349364953241133i, 2.1028962986076503e-05+0.000735803180165176i, 2.2105881774023284e-05+0.0007365826661086842i, 2.195269216857454e-05+0.0007370666351362634i, 2.2944142536568783e-05+0.000738127734544367i, 2.2594225296326463e-05+0.0007379654494961671i, 2.2991647784206674e-05+0.0007395610917658905i, 2.3061333198931392e-05+0.0007392509647770023i, 2.2895663522589002e-05+0.0007392496570797655i, 2.3522359385112018e-05+0.0007401551101051218i, 2.3758774110465428e-05+0.0007409229758497907i, 2.4074391877354853e-05+0.0007408003808736765i, 2.369724972829126e-05+0.0007419127553707i, 2.4196489534957747e-05+0.0007416263905465133i, 2.4788286637432465e-05+0.0007423997071167373i, 2.437100659110085e-05+0.0007423726956851667i, 2.4436145178907698e-05+0.0007433577459097762i, 2.4630974178041407e-05+0.0007429029540941432i, 2.5085569212968363e-05+0.0007433307970902484i, 2.4928911496653477e-05+0.0007437865358384905i, 2.4997082296247526e-05+0.0007440816556151765i, 2.481615794105754e-05+0.000744689260767696i, 2.4256112896251368e-05+0.0007446534419087711i, 2.519658215377437e-05+0.0007455103199150154i, 2.5386526220959067e-05+0.0007450821310619119i, 2.5195390736045592e-05+0.0007456887582739535i, 2.491297345208157e-05+0.0007453899491571836i, 2.490013440547585e-05+0.0007459573174257771i, 2.473084575305942e-05+0.0007462436035376812i, 2.5244618113013167e-05+0.0007469393026418149i, 2.519002518212992e-05+0.0007468684747063853i, 2.5127560426703364e-05+0.0007468887240373331i, 2.5077375979938654e-05+0.000747052914876855i, 2.429082024234024e-05+0.0007474931306089232i, 2.478161100105928e-05+0.0007475443788641105i]
  out "Error Out":errorcluster
  in  "Error In":errorcluster
  in  "cursor bracket: fit boundaries":T8={"left"=1991588.8394960614, "right "=1997520.3804847973, "center"=1994554.6099904294, "window"=5931.540988735925, "cursors"=[3, 4, 5], "relative"=1, "absolute"=4, "fixed vertical offset"=0.0, "vertical offset"=0.0, "skew"=0.0, "default window frac"=0.1, "kind"=enum."symmetric", "skew.left"=0.5, "skew.right"=0.5, "Plot ref"=refnum, "wing order"=enum."forw"}
  in  "scan monitor control":T9={"gamma acc. frac. - min "=0.3, "gamma acc frac.. - max"=3.0, "peak acc. fraction (af)"=5.0, "min peak acc. window (kHz)"=0.5, "use"=enum."fraction", "abs gamma min(kHz)"=0.005, "abs gamma max(kHz)"=5.0, "# points"=5, "gamma-factor (fa)"=2.0, "interpolate"=enum."line", "init"=TRUE, "Unique strike parameters"=TRUE, "max peak acc. window (kHz)"=10.0, "spacing factor"=1.5, "iterate #"=1, "overwrite ctl?"=FALSE, "write _m files?"=FALSE, "max slope (kHz/sweep)"=0.5, "funnel state"=enum."funnel open"}
  in  "Update system parameters":bool
  in  "parameters: complex fit":T10={"main VI path"=path "", "scale factor"=3.0, "# of grid points"=200, "parameters: wavepacket"={"R"=0.5, "wave number"=22.0, "delta k"=7.0, "radii vector"=[], "radial section"=[], "wave vector"=22.0, "wavepacket is"=TRUE}, "span"=0.27789, "interference ?"=enum."cp z center", "filter method"=enum."three"} {"span" min=0.0 max=0.5 step=1e-05 scale=0.0001..0.5 scale format="%#_5f"; "parameters: wavepacket"."delta k" format="%#_3f"; "parameters: wavepacket"."wave number" format="%#_3f"; "parameters: wavepacket"."R" format="%#_3f"}
  in  "cursor bracket: circle window":T8={"left"=1993181.8368605364, "right "=1995927.3831203224, "center"=1994554.6099904294, "window"=2745.5462597861706, "cursors"=[0, 1, 2], "relative"=1, "absolute"=1, "fixed vertical offset"=0.0, "vertical offset"=0.0, "skew"=0.0, "default window frac"=0.1, "kind"=enum."symmetric", "skew.left"=0.5, "skew.right"=0.5, "Plot ref"=refnum, "wing order"=enum."forw"}
  in  "Tab : parameters":enum32{"Page 1"}(tab)
  out "VKey":T13
  out "Char":i16=54
  # "three strikes"
  # "search window"
  # "linear extrapolation"
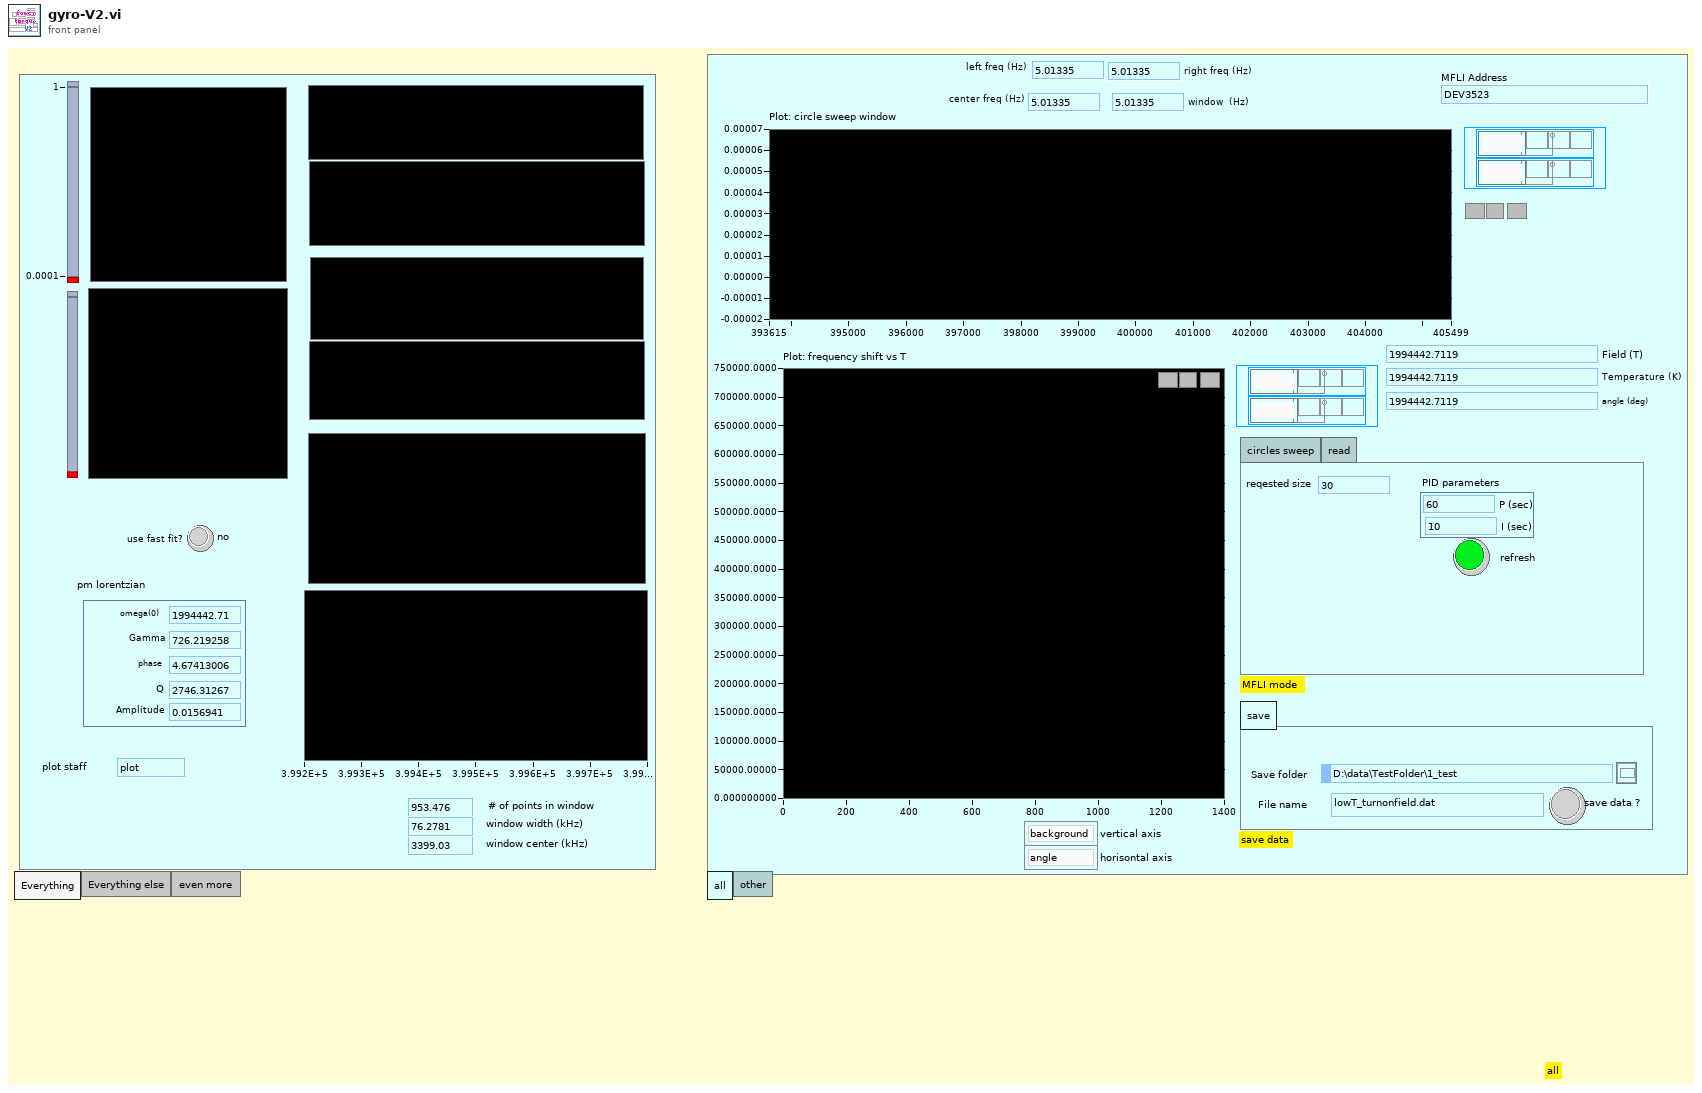
[diagram p1: front panel]
types:
  T1 = typedef "pid -- parameters.ctl" = cluster{"P (sec)":dbl, "I (sec)":dbl}
  T2 = enum16{"frequency", "gamma", "phase", "background"}
  T3 = typedef "agregator -- action.ctl" = enum16{"append", "interpolate", "empty!", "force", "init", "scale", "read last"}
  T4 = enum32{"Everything", "Everything else", "even more "}
  T5 = cluster{"omega out":dbl[], "win omega out":dbl[]}
  T6 = typedef "lorentzian.ctl" = cluster{"Amplitude":dbl, "omega(0)":dbl, "Gamma":dbl, "phase":dbl, "Q":dbl, "Norm  Ampl":dbl, "z (inf)":cdb, "4corners":T7}
  T7 = typedef "circle corners.ctl" = cluster{"z (-pi/2)":cdb, "z(inf)":cdb, "z (pi/2)":cdb, "z center":cdb, "z(0)":cdb, "radius":dbl}
  T8 = typedef "cursor winow.ctl" = cluster{"left":dbl, "right ":dbl, "center":dbl, "window":dbl, "cursors":i32[], "relative":i32, "absolute":i32, "fixed vertical offset":dbl, "vertical offset":dbl, "skew":dbl, "default window frac":dbl, "kind":enum16{"symmetric", "skewed", "fancy"}, "skew.left":dbl, "skew.right":dbl, "Plot ref":refnum<vi>, "wing order":enum16{"forw", "back"}}
  T9 = typedef "parameters -- scan monitor control.ctl" = cluster{"gamma acc. frac. - min ":dbl, "gamma acc frac.. - max":dbl, "peak acc. fraction (af)":dbl, "min peak acc. window (kHz)":dbl, "use":enum16{"window", "fraction"}, "abs gamma min(kHz)":dbl, "abs gamma max(kHz)":dbl, "# points":i32, "gamma-factor (fa)":dbl, "interpolate":enum16{"line", "last"}, "init":bool, "Unique strike parameters":bool, "max peak acc. window (kHz)":dbl, "spacing factor":dbl, "iterate #":i32, "overwrite ctl?":bool, "write _m files?":bool, "max slope (kHz/sweep)":dbl, "funnel state":enum16{"funnel open", "funnel closed"}}
  T10 = typedef "peak -- parameters -- complex fit.ctl" = cluster{"main VI path":path, "scale factor":dbl, "# of grid points":i32, "parameters: wavepacket":T11, "span":dbl, "interference ?":enum16{"cp z center", "pm zcenter", "fancy"}, "filter method":T12}
  T11 = typedef "wavepacket.ctl" = cluster{"R":dbl, "wave number":dbl, "delta k":dbl, "radii vector":dbl[], "radial section":cdb[], "wave vector":dbl, "wavepacket is":bool}
  T12 = typedef "filter method control.ctl" = enum16{"four", "five", "one", "two", "three", "zero", "minus one", "minus two"}
  T13 = typedef "eventvkey.ctl" = enum16{"ASCII", "Enter", "Return", "Shift", "Ctrl", "Alt", "Cmd", "Opt", "Caps", "NumLock", "Clear", "Break", "Up", "Down", "Left", "Right", "Insert", "Delete", "Home", "End", "PageUp", "PageDown", "Escape", "Help", "Pause", "ScrollLock", "F1", "F2", "F3", "F4", "F5", "F6", "F7", "F8", "F9", "F10", "F11", "F12", "F13", "F14", "F15", "F16", "F17", "F18", "F19", "F20", "F21", "F22", "F23", "F24", "Play", "VolumeUp", "VolumeDown", "Mute", "Two Byte Char"}
  T14 = typedef "MFLI controller action.ctl" = enum16{"Initialize", "Scan frequency", "open", "close", "read", "circle PLL"}
  T15 = typedef "cursor window action.ctl" = enum16{"balance", "h. offset change", "cursor moves", "change center", "change window", "init", "check", "reset", "set y to middle", "idle", "-write all Y", "-write left.X", "-write center.X", "-write right.X", "-write all X", "-change center", "-change window", "-change skew", "-read cursor 2", "-read cursor 1", "-read cursor 0", "-read all cursors", "-reset", "-read plot scale", "-set y to middle", "-Q: center.Y is visible", "-Q: window is visible", "-parse center.Y", "-right left from center", "-left move", "-right move", "-set center.Y", "-empty", "-set cursors to default", "-check", "-write center.Y", "-copy cursor 1", "-copy cursor 0", "-copy cursor 2", "move right", "move left", "shrink", "broaden", "skew up", "skew down", "-write plot scale", "zoom X", "change cen&win", "zoom to all data", "color--red", "color--green", "color--yellow", "read", "zoom out", "zoom in", "slide right", "slide left"}
  T16 = typedef "plot refs -- filter related.ctl" = cluster{"Plot: complex plane - filter":refnum<vi>, "Plot: dz/domega":refnum<vi>, "Plot: fragment filter":refnum<vi>, "Plot: win omega":refnum<vi>, "Plot: phase":refnum<vi>, "Plot: phase around center":refnum<vi>, "Plot: complex plane":refnum<vi>, "Plot: fragment":refnum<vi>}
  T17 = typedef "sweep parameters.ctl" = cluster{"scan type":enum16{"linear", "arctan"}, "N":i64, "cursor window":T8}
  T18 = typedef "cursor action.ctl" = enum16{"range", "read", "write", "check", "zoom out", "smart zoom out"}
  T19 = typedef "KM_file -- read-write control.ctl" = enum16{"read", "write all", "append one line"}
  T20 = typedef "four-corner circle transformation.ctl" = enum16{"z(c) z(inf)", "z(c) z(zero)", "fix phase", "calculate lorentzian", "z(0) z(+-pi/2)", "shift to zcenter", "to  canonical", "get canonical phase"}
  T21 = typedef "interpolation state - real.ctl" = cluster{"requested size":i32, "Array":dbl[], "actual number of elements":i32}
  T22 = typedef "interpolation state - complex.ctl" = cluster{"requested size":i32, "Array":cdb[], "actual number of elements":i32}
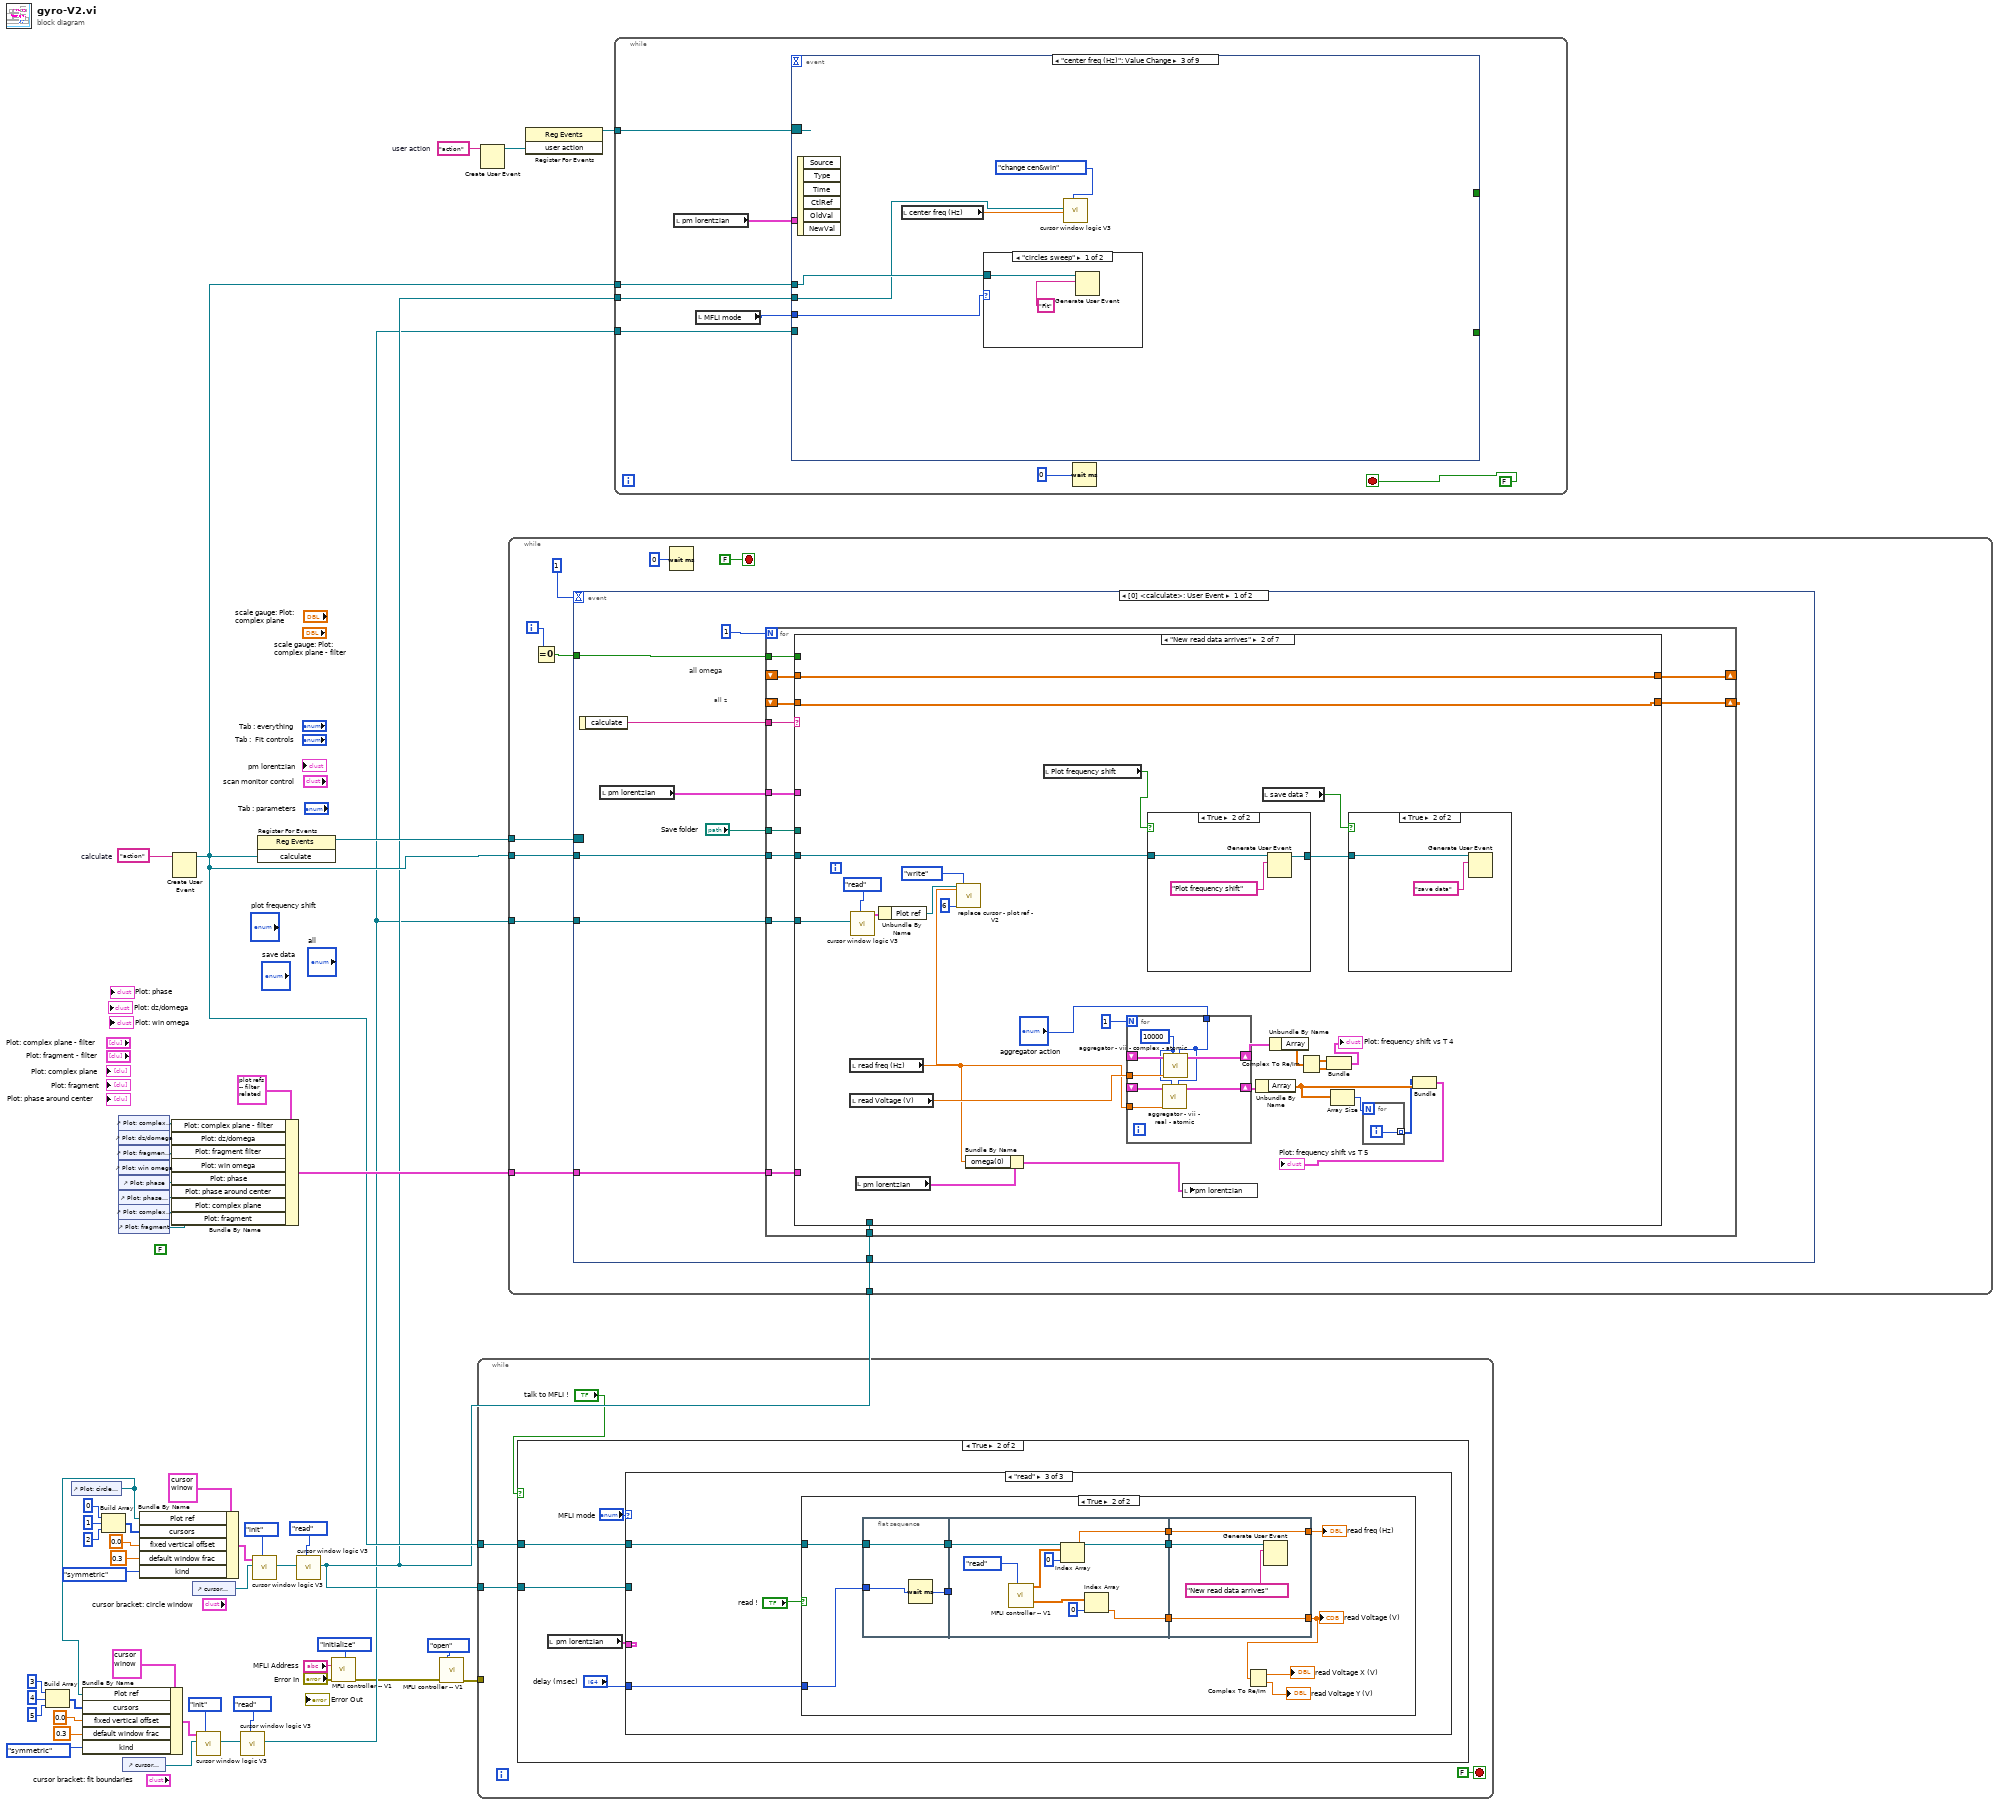
[diagram p0: block diagram]
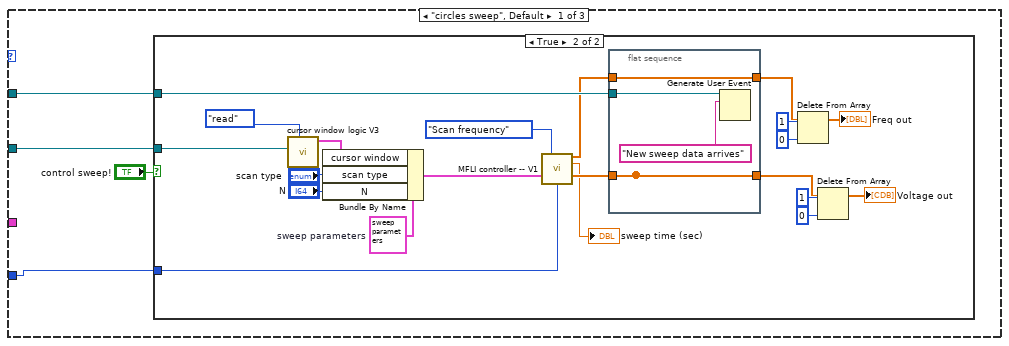
[diagram p3: hidden frame]
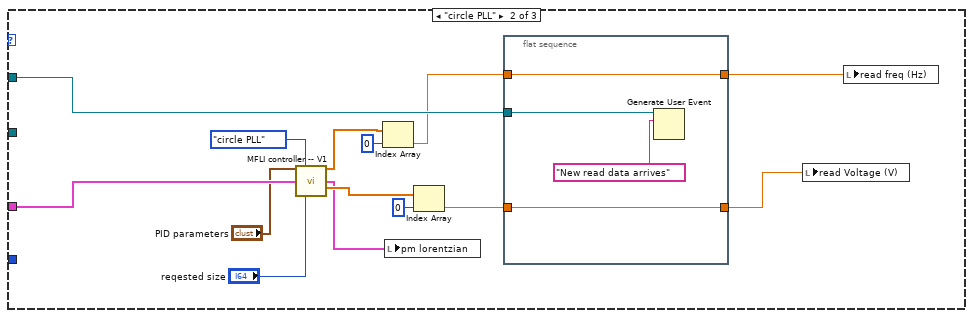
[diagram p5: hidden frame]
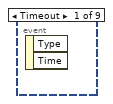
[diagram p7: hidden frame]
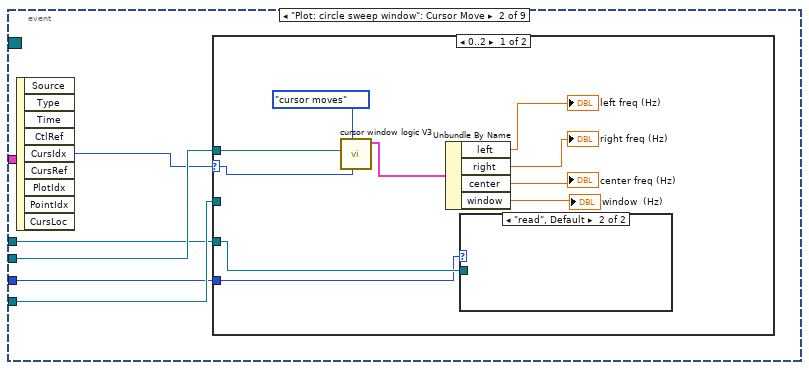
[diagram p8: hidden frame]
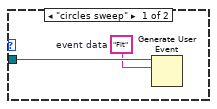
[diagram p9: hidden frame]
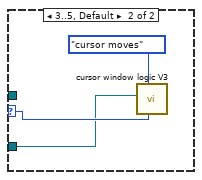
[diagram p10: hidden frame]
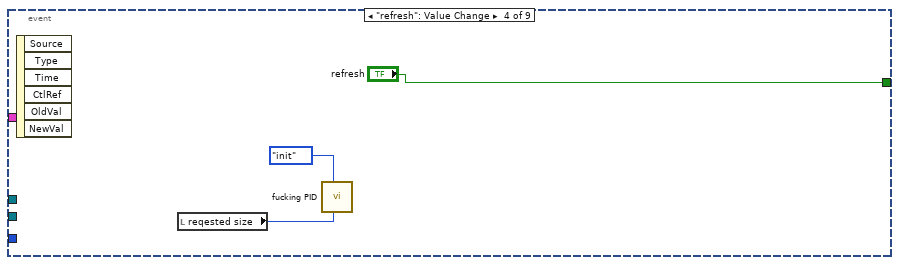
[diagram p12: hidden frame]
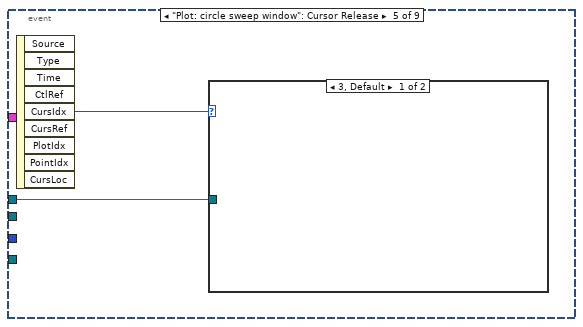
[diagram p13: hidden frame]
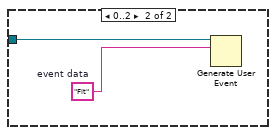
[diagram p14: hidden frame]
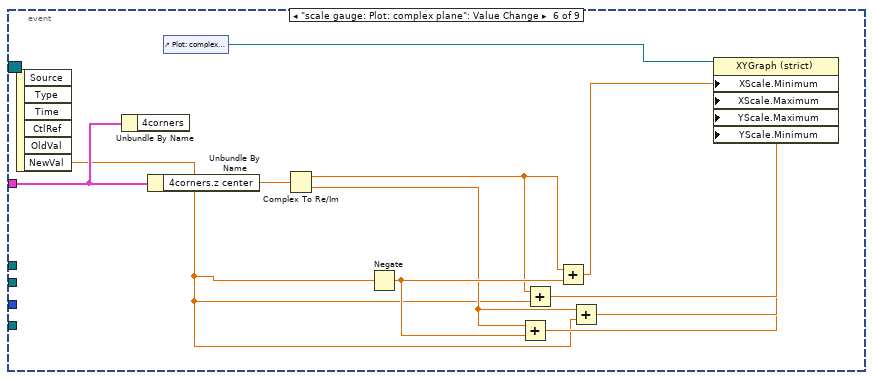
[diagram p15: hidden frame]
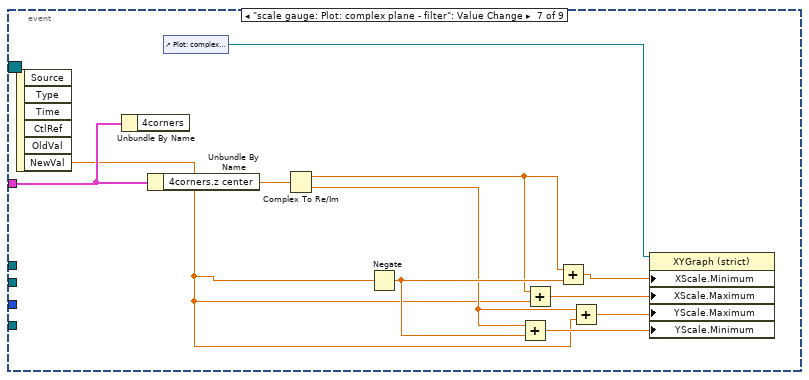
[diagram p16: hidden frame]
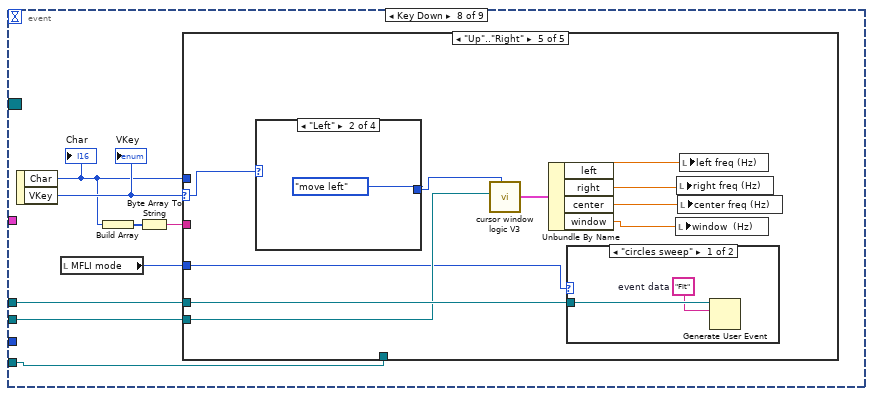
[diagram p17: hidden frame]
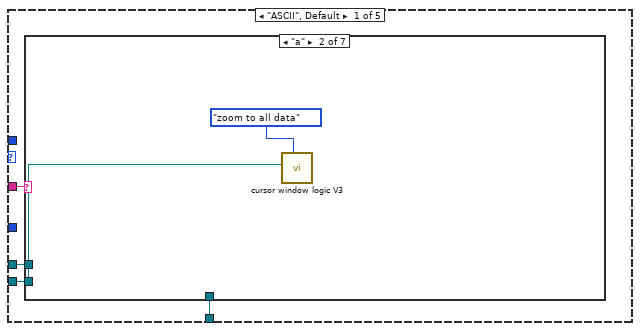
[diagram p18: hidden frame]
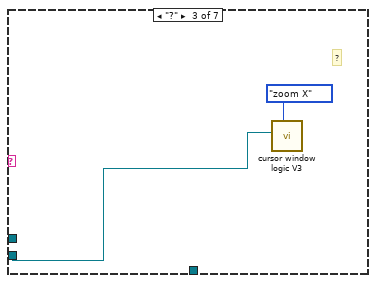
[diagram p20: hidden frame]
diagram:
  w48 = "action"  # user action
  w50 = "action"  # calculate
  (unwired) FALSE
  n1 = Build Array(3, 4, 5) -> (w18:i32[])
  n2 = control-ref of="Plot: circle sweep window"() -> (w5:refnum<vi>)
  n3 = Bundle By Name(cluster=T8 {"left"=0.0, "right "=0.0, "center"=0.0, "window"=0.0, "cursors"=[], "relative"=0, "absolute"=0, "fixed vertical offset"=0.0, "vertical offset"=0.0, "skew"=0.0, "default window frac"=0.0, "kind"=enum."symmetric", "skew.left"=0.0, "skew.right"=0.0, "Plot ref"=refnum, "wing order"=enum."forw"} ("cursor bracket: All, data window"), "Plot ref"=w5, "cursors"=w18, "fixed vertical offset"=0.0, "default window frac"=0.3 ("fixed vertical offset"), "kind"=enum16{"symmetric", "skewed", "fancy"}."symmetric") -> (w10:T8)
  n4 = Build Array(0, 1, 2) -> (w35:i32[])
  n5 = control-ref of="Plot: complex plane - filter"() -> (w45:refnum<vi>)
  n6 = control-ref of="Plot: dz/domega"() -> (w44:refnum<vi>)
  n7 = control-ref of="Plot: fragment - filter"() -> (w43:refnum<vi>)
  n8 = control-ref of="Plot: win omega"() -> (w42:refnum<vi>)
  n9 = control-ref of="Plot: phase"() -> (w41:refnum<vi>)
  n10 = control-ref of="Plot: phase around center"() -> (w39:refnum<vi>)
  n11 = control-ref of="Plot: complex plane"() -> (w38:refnum<vi>)
  n12 = control-ref of="Plot: fragment"() -> (w37:refnum<vi>)
  n13 = control-ref of="cursor bracket: fit boundaries"() -> (w6:refnum<vi>)
  n14 = Bundle By Name(cluster=T8 {"left"=0.0, "right "=0.0, "center"=0.0, "window"=0.0, "cursors"=[], "relative"=0, "absolute"=0, "fixed vertical offset"=0.0, "vertical offset"=0.0, "skew"=0.0, "default window frac"=0.0, "kind"=enum."symmetric", "skew.left"=0.0, "skew.right"=0.0, "Plot ref"=refnum, "wing order"=enum."forw"} ("cursor bracket: All, data window"), "Plot ref"=w5, "cursors"=w35, "fixed vertical offset"=0.0, "default window frac"=0.3 ("fixed vertical offset"), "kind"=enum16{"symmetric", "skewed", "fancy"}."symmetric") -> (w27:T8)
  n15 = Bundle By Name(cluster=T16 {"Plot: complex plane - filter"=refnum, "Plot: dz/domega"=refnum, "Plot: fragment filter"=refnum, "Plot: win omega"=refnum, "Plot: phase"=refnum, "Plot: phase around center"=refnum, "Plot: complex plane"=refnum, "Plot: fragment"=refnum} ("plots: filter related"), "Plot: complex plane - filter"=w45, "Plot: dz/domega"=w44, "Plot: fragment filter"=w43, "Plot: win omega"=w42, "Plot: phase"=w41, "Plot: phase around center"=w39, "Plot: complex plane"=w38, "Plot: fragment"=w37) -> (w40:T16)
  n16 = Create User Event(user event datatype=w50) -> (user event=w36:refnum<user-event>)  [unwired: 1 in, 1 out]
  n17 = control-ref of="cursor bracket: circle window"() -> (w26:refnum<vi>)
  n18 = call "cursor window logic V3.vi"("cursor window action"=cursor_window_action."init", "cursor window in"=w6, "cursor window init"=w10) -> ("cursor window out"=w8:refnum<vi>)  [unwired: 7 in, 1 out]
  n19 = call "cursor window logic V3.vi"("cursor window action"=cursor_window_action."read", "cursor window in"=w8) -> ("cursor window out"=w4:refnum<vi>)  [unwired: 8 in, 1 out]
  n20 = call "cursor window logic V3.vi"("cursor window action"=cursor_window_action."init", "cursor window in"=w26, "cursor window init"=w27) -> ("cursor window out"=w24:refnum<vi>)  [unwired: 7 in, 1 out]
  n21 = register-events(w36) -> (reference out=w51:refnum<event-registration>)  [unwired: 2 in, 1 out]
  n22 = call "cursor window logic V3.vi"("cursor window action"=cursor_window_action."read", "cursor window in"=w24) -> ("cursor window out"=w22:refnum<vi>)  [unwired: 8 in, 1 out]
  n23 = call "MFLI controller -- V1.vi"("MFLI controller action"=MFLI_controller_action."Initialize", "Address"="MFLI Address", "Error In"="Error In") -> ("Error Out"=w2:errorcluster)  [unwired: 8 in, 4 out]
  n24 = call "MFLI controller -- V1.vi"("MFLI controller action"=MFLI_controller_action."open", "Error In"=w2) -> ("Error Out"=w1:errorcluster)  [unwired: 9 in, 4 out]
  n25 = while {
    tunnel: w36 -> [w55]
    tunnel: w22 -> [w53]
    tunnel: w1 -> [_]
    stop <- FALSE stop-if-true
    n26 = case shown="True" "talk to MFLI !" {
      tunnel: w55 -> [_ w60]
      tunnel: w53 -> [_ w59]
      frame False {
      }
      frame True {
        n27 = local read "pm lorentzian"() -> (w57:T6)
        n28 = case shown="\"read\"" "MFLI mode" {
          tunnel: w60 -> [w64 w96 w110]
          tunnel: w59 -> [w63 _ _]
          tunnel: w57 -> [_ w102 _]
          tunnel: "delay (msec)" -> [w61 _ w108]
          frame "circles sweep", Default {
            n29 = case shown="True" "control sweep!" {
              tunnel: w64 -> [_ w85]
              tunnel: w63 -> [_ w84]
              tunnel: w61 -> [_ w65]
              frame False {
              }
              frame True {
                w79 = T17 {"scan type"=enum."linear", "N"=-1, "cursor window"={"left"=2378.60310421286, "right "=2421.6740576496672, "center"=2421.6740576496672, "window"=2421.6740576496672, "cursors"=[], "relative"=0, "absolute"=0, "fixed vertical offset"=2421.6740576496672, "vertical offset"=2421.6740576496672, "skew"=2421.6740576496672, "default window frac"=2421.6740576496672, "kind"=enum."skewed", "skew.left"=2421.6740576496672, "skew.right"=2421.6740576496672, "Plot ref"=refnum, "wing order"=enum."back"}}  # sweep parameters
                n30 = call "cursor window logic V3.vi"("cursor window action"=cursor_window_action."read", "cursor window in"=w84) -> ("cursor window out"=w77:T8)  [unwired: 8 in, 1 out]
                n31 = Bundle By Name(cluster=w79, "cursor window"=w77, "scan type"="scan type", "N"="N") -> (w75:T17)
                n32 = call "MFLI controller -- V1.vi"("MFLI controller action"=MFLI_controller_action."Scan frequency", "sweep parameters"=w75, "delay (msec)"=w65) -> ("Freq out (Hz)"=w81:dbl[], "sweep time"=→"sweep time (sec)":dbl, "Voltage out (V)"=w80:cdb[])  [unwired: 8 in, 2 out]
                n33 = flat-sequence {
                  tunnel: w81 -> [w89]
                  tunnel: [w89] -> w71
                  tunnel: w85 -> [w87]
                  tunnel: [w86] -> _
                  tunnel: w80 -> [w86]
                  tunnel: [w86] -> w66
                  frame #0 {
                    n34 = Generate User Event(user event=w87, event data cluster="New sweep data arrives" ("event data")) -> ()  [unwired: 2 in, 2 out]
                  }
                }
                n35 = Delete From Array(array=w71, length=1, index=0) -> (array with subset deleted=→"Freq out":dbl[])  [unwired: 1 out]
                n36 = Delete From Array(array=w66, length=1, index=0) -> (array with subset deleted=→"Voltage out":cdb[])  [unwired: 1 out]
              }
            }
          }
          frame "circle PLL" {
            n37 = call "MFLI controller -- V1.vi"("PID parameters"="PID parameters", "MFLI controller action"=MFLI_controller_action."circle PLL", "lorentzian in"=w102, "reqested size"="reqested size") -> ("Freq out (Hz)"=w98:dbl[], "lorentzian out"=w91:T6, "Voltage out (V)"=w97:cdb[])  [unwired: 7 in, 2 out]
            n38 = Index Array(array=w98, index=0) -> (element=w94:dbl)
            n39 = local write "pm lorentzian"(w91) -> ()
            n40 = Index Array(array=w97, index=0) -> (element=w92:cdb)
            n41 = flat-sequence {
              tunnel: w96 -> [w106]
              tunnel: [w105] -> w95
              tunnel: w94 -> [w105]
              tunnel: [w104] -> w93
              tunnel: w92 -> [w104]
              frame #0 {
                n42 = Generate User Event(user event=w106, event data cluster="New read data arrives" ("event data")) -> ()  [unwired: 2 in, 2 out]
              }
            }
            n43 = local write "read Voltage (V)"(w93) -> ()
            n44 = local write "read freq (Hz)"(w95) -> ()
          }
          frame "read" {
            n45 = case shown="True" "read !" {
              tunnel: w110 -> [_ w121]
              tunnel: w108 -> [_ w115]
              frame False {
              }
              frame True {
                n46 = flat-sequence {
                  tunnel: w121 -> [w124]
                  tunnel: [w124] -> w116
                  tunnel: w115 -> [w123]
                  tunnel: [w122] -> w114
                  tunnel: [w125] -> w119
                  tunnel: [w132] -> w118
                  tunnel: [w126] -> w117
                  tunnel: w116 -> [w132]
                  tunnel: w114 -> [_]
                  tunnel: [w136] -> w120
                  tunnel: [w133] -> w113
                  tunnel: w119 -> [w136]
                  tunnel: w118 -> [w134]
                  tunnel: w117 -> [w133]
                  frame #0 {
                    n47 = Wait (ms)(milliseconds to wait=w123) -> (millisecond timer value=w122:u32)
                  }
                  frame #1 {
                    n48 = call "MFLI controller -- V1.vi"("MFLI controller action"=MFLI_controller_action."read") -> ("Freq out (Hz)"=w128:dbl[], "Voltage out (V)"=w130:cdb[])  [unwired: 10 in, 3 out]
                    n49 = Index Array(array=w128, index=0) -> (element=w125:dbl)
                    n50 = Index Array(array=w130, index=0) -> (element=w126:cdb)
                  }
                  frame #2 {
                    n51 = Generate User Event(user event=w134, event data cluster="New read data arrives" ("event data")) -> ()  [unwired: 2 in, 2 out]
                  }
                }
                n52 = Complex To Re/Im(x + iy=w113) -> (x=→"read Voltage X (V)":dbl, y=→"read Voltage Y (V)":dbl)
                "read freq (Hz)" <- w120
                "read Voltage (V)" <- w113
              }
            }
          }
        }
      }
    }
  }
  n53 = Create User Event(user event datatype=w48) -> (user event=w47:refnum<user-event>)  [unwired: 1 in, 1 out]
  n54 = while {
    tunnel: w51 -> [w146]
    tunnel: w36 -> [w144]
    tunnel: w40 -> [w140]
    tunnel: w22 -> [w138]
    tunnel: w4 -> [w137]
    i -> [w141]
    stop <- FALSE stop-if-true
    n55 = Equal To 0?(x=w141) -> (x = 0?=w139:bool)
    n56 = event shown="[0] <calculate>: User Event" {
      selector: w146 -> [_ _]
      dyn-events: _ -> [_ _]
      timeout: 1 -> [_ _]
      tunnel: w144 -> [w154 _]
      tunnel: w140 -> [w151 _]
      tunnel: w139 -> [w150 _]
      tunnel: w138 -> [w149 _]
      tunnel: w137 -> [w147 _]
      event User Event {
        # "all z"
        # "all omega"
        n57 = event-data() -> ("calculate"=w155:string)  [unwired: 1 in]
        n58 = local read "pm lorentzian"() -> (w148:T6)
        n59 = for {
          N: 1 -> [_]
          tunnel: w155 -> [w167]
          tunnel: w154 -> [w166]
          shift-right: [w160] -> _
          shift-left: _ -> [w165]
          shift-right: [w159] -> _
          shift-left: _ -> [w164]
          tunnel: "Save folder" -> [w163]
          tunnel: w151 -> [w162]
          tunnel: w150 -> [w161]
          tunnel: w149 -> [w158]
          tunnel: w148 -> [w157]
          tunnel: w147 -> [w156]
          n60 = case shown="\"New read data arrives\"" w167 {
            tunnel: w166 -> [w178 w217 _ _ _ _ _]
            tunnel: w165 -> [_ w216 w271 w290 w310 w326 w354]
            tunnel: w164 -> [_ w215 w270 w289 w309 w323 w353]
            tunnel: w163 -> [_ _ _ w285 w307 _ _]
            tunnel: w162 -> [_ _ _ _ _ w330 _]
            tunnel: w161 -> [_ _ _ _ _ _ _]
            tunnel: [w172 w216 w271 w290 w310 w326 w354] -> w160
            tunnel: [w168 w215 w270 w289 w309 w323 w353] -> w159
            tunnel: w158 -> [_ _ _ _ w308 w328 _]
            tunnel: w157 -> [_ _ w256 w284 w306 _ _]
            tunnel: w156 -> [_ w214 _ _ w299 _ _]
            frame "New sweep data arrives" {
              n61 = Generate User Event(user event=w178, event data cluster="Fit" ("event data")) -> (user event out=w175:refnum<user-event>)  [unwired: 2 in, 1 out]
              n62 = case shown="True" "Auto-update sweep window!" {
                tunnel: w175 -> [w185 w187]
                tunnel: [w185 w186] -> w174
                frame False {
                }
                frame True {
                  n63 = Generate User Event(user event=w187, event data cluster="Update range" ("event data")) -> (user event out=w186:refnum<user-event>)  [unwired: 2 in, 1 out]
                }
              }
              n64 = local read "Voltage out"() -> (w168:cdb[])
              n65 = local read "Freq out"() -> (w172:dbl[])
              n66 = case shown="True" "Plot frequency shift" {
                tunnel: w174 -> [w189 w191]
                tunnel: [w189 w190] -> w170
                frame False {
                }
                frame True {
                  n67 = Generate User Event(user event=w191, event data cluster="Plot frequency shift" ("event data")) -> (user event out=w190:refnum<user-event>)  [unwired: 2 in, 1 out]
                }
              }
              n68 = Complex To Re/Im(x + iy=w168) -> (x=w181:dbl[], y=w180:dbl[])
              n69 = Bundle("Freq out"=w172, w181) -> (w182:cluster{"Freq out":dbl[], dbl[]})  [unwired: 1 in]
              n70 = Bundle("Freq out"=w172, w180) -> (w179:cluster{"Freq out":dbl[], dbl[]})  [unwired: 1 in]
              n71 = Build Array(w182, w179) -> (→"Plot: circle sweep window":cluster{"Freq out":dbl[], dbl[]}[])
              n72 = case shown="True" "save data ?" {
                tunnel: w170 -> [_ w183]
                frame False {
                }
                frame True {
                  n73 = Generate User Event(user event=w183, event data cluster="save data" ("event data")) -> ()  [unwired: 2 in, 2 out]
                }
              }
            }
            frame "New read data arrives" {
              n74 = local read "read freq (Hz)"() -> (w194:dbl)
              n75 = local read "read Voltage (V)"() -> (w197:cdb)
              n76 = call "cursor window logic V3.vi"("cursor window action"=cursor_window_action."read", "cursor window in"=w214) -> ("cursor window out"=w212:T8)  [unwired: 8 in, 1 out]
              n77 = local read "pm lorentzian"() -> (w195:T6)
              n78 = Unbundle By Name(w212) -> ("Plot ref"=w211:refnum<vi>)
              n79 = call "replace cursor - plot ref - V2.vi"("Plot ref in"=w211, "new X"=w194, "cursor index"=6, "cursor action"=cursor_action."write") -> ()  [unwired: 13 in, 3 out]
              n80 = Bundle By Name(cluster=w195, "omega(0)"=w194) -> (w193:T6)
              n81 = local read "Plot frequency shift"() -> (w218:bool)
              n82 = for {
                N: 1 -> [_]
                shift-right: [w229] -> w208
                shift-left: _ -> [w228]
                tunnel: w197 -> [w227]
                tunnel: w194 -> [w226]
                shift-right: [w224] -> w206
                shift-left: _ -> [w225]
                tunnel: "aggregator action" -> [w222]
                w223 = 10000
                n83 = call "aggregator - vii - real - atomic.vi"("aggregator action"=w222, "requested size"=w223, "number"=w226, "state IN"=w225) -> ("state OUT"=w224:T21)  [unwired: 4 in, 3 out]
                n84 = call "aggregator - vii - complex - atomic.vi"("aggregator action"=w222, "requested size"=w223, "number"=w227, "state IN"=w228) -> ("state OUT"=w229:T22)  [unwired: 4 in, 3 out]
              }
              n85 = case shown="True" w218 {
                tunnel: w217 -> [w232 w234]
                tunnel: [w232 w233] -> w220
                frame False {
                }
                frame True {
                  n86 = Generate User Event(user event=w234, event data cluster="Plot frequency shift" ("event data")) -> (user event out=w233:refnum<user-event>)  [unwired: 2 in, 1 out]
                }
              }
              n87 = local write "pm lorentzian"(w193) -> ()
              n88 = Unbundle By Name(w206) -> ("Array"=w204:dbl[])
              n89 = local read "save data ?"() -> (w219:bool)
              n90 = Unbundle By Name(w208) -> ("Array"=w201:cdb[])
              n91 = Complex To Re/Im(x + iy=w201) -> (x=w200:dbl[], y=w199:dbl[])
              n92 = Bundle(w200, w199) -> (→"Plot: frequency shift vs T 4":cluster{dbl[], dbl[]})  [unwired: 1 in]
              n93 = Array Size(array=w204) -> (size(s)=w205:i32)
              n94 = case shown="True" w219 {
                tunnel: w220 -> [_ w230]
                frame False {
                }
                frame True {
                  n95 = Generate User Event(user event=w230, event data cluster="save data" ("event data")) -> ()  [unwired: 2 in, 2 out]
                }
              }
              n96 = for {
                N: w205 -> [_]
                tunnel: [w221] -> w203 mode=indexing
                i -> [w221]
              }
              n97 = Bundle(w203, "Array"=w204) -> (→"Plot: frequency shift vs T 5":cluster{i32[], "Array":dbl[]})  [unwired: 1 in]
            }
            frame "Plot frequency shift" {
              (unwired) T2."background"
              (unwired) enum16{"Time", "temperature", "field", "angle"}."angle"
              w238 = 1000000 ("requested size")
              # "omega (Hz)"
              # "time (min)"
              n98 = Unbundle By Name(w256) -> ("omega(0)"=w261:dbl, "Gamma"=w260:dbl, "phase"=w242:dbl, "z (inf)"=w240:cdb)
              n99 = call <vilib>:"High Resolution Relative Seconds.vi"() -> ("relative seconds"=w262:dbl)
              n100 = Divide(x=w262, y=60) -> (x/y=w264:dbl)
              n101 = Complex To Polar(r * e^(i*theta)=w240) -> (r=w239:dbl)  [unwired: 1 out]
              n102 = Multiply(x="plot length (min)", y=60) -> (x*y=w266:dbl)
              n103 = call "fancy torque read T .vi"() -> ("angle"=w248:dbl, "field"=w249:dbl, "temperature"=w255:dbl)  [unwired: 8 in, 1 out]
              n104 = Divide(x=w266, y="aggregate every # sec") -> (x/y=w265:dbl)
              n105 = Round Toward +Infinity(x=w265) -> (ceil(x): smallest int >= x=w268:dbl)
              n106 = call "switch - C.vi"("switch"=TRUE) -> ("result"=w236:bool)  [unwired: 10 in]
              n107 = To Long Integer(number=w268) -> ()  [unwired: 1 out]
              n108 = call "aggregator - v - real.vi"("number"=w239, "init?"=w236, "requested size"=w238) -> ("Array"=w237:dbl[])  [unwired: 6 in, 2 out]
              n109 = call "aggregator - v - real.vi"("number"=w242, "init?"=w236, "requested size"=w238) -> ("Array"=w241:dbl[])  [unwired: 6 in, 2 out]
              n110 = call "aggregator - v - real.vi"("number"=w264, "init?"=w236, "requested size"=w238) -> ("Array"=w251:dbl[])  [unwired: 6 in, 2 out]
              n111 = call "aggregator - v - real.vi"("number"=w261, "init?"=w236, "requested size"=w238) -> ("Array"=w244:dbl[])  [unwired: 6 in, 2 out]
              n112 = call "aggregator - v - real.vi"("number"=w260, "init?"=w236, "requested size"=w238) -> ("Array"=w243:dbl[])  [unwired: 6 in, 2 out]
              n113 = call "aggregator - v - real.vi"("number"=w255, "init?"=w236, "requested size"=w238) -> ("Array"=w253:dbl[])  [unwired: 6 in, 2 out]
              n114 = call "aggregator - v - real.vi"("number"=w249, "init?"=w236, "requested size"=w238) -> ("Array"=w250:dbl[])  [unwired: 6 in, 2 out]
              n115 = call "aggregator - v - real.vi"("number"=w248, "init?"=w236, "requested size"=w238) -> ("Array"=w247:dbl[])  [unwired: 6 in, 2 out]
              n116 = case shown="\"angle\"" "horisontal axis" {
                tunnel: w253 -> [_ w277 _ _]
                tunnel: [w276 w277 w278 w279] -> w252
                tunnel: w251 -> [w276 _ _ _]
                tunnel: w250 -> [_ _ w278 _]
                tunnel: w247 -> [_ _ _ w279]
                frame "Time", Default {
                }
                frame "temperature" {
                }
                frame "field" {
                }
                frame "angle" {
                }
              }
              n117 = case shown="\"gamma\"" "vertical axis" {
                tunnel: w243 -> [_ w273 _ _]
                tunnel: [w272 w273 w274 w275] -> w245
                tunnel: w244 -> [w272 _ _ _]
                tunnel: w241 -> [_ _ w274 _]
                tunnel: w237 -> [_ _ _ w275]
                frame "frequency", Default {
                }
                frame "gamma" {
                }
                frame "phase" {
                }
                frame "background" {
                }
              }
              n118 = Bundle("Array"=w252, "Array"=w245) -> (→"Plot: frequency shift vs T":cluster{"Array":dbl[], "Array":dbl[]})  [unwired: 1 in]
            }
            frame "save data" {
              n119 = call <vilib>:"High Resolution Relative Seconds.vi"() -> ("relative seconds"=w283:dbl)
              n120 = Unbundle By Name(w284) -> ()  [unwired: 2 out]
              n121 = call "fancy torque read T .vi"() -> ("angle"=w281:dbl, "field"=w280:dbl, "temperature"=w282:dbl)  [unwired: 8 in, 1 out]
              "Field (T)" <- w280
              n122 = call "switch - C.vi"("switch"=TRUE) -> ()  [unwired: 10 in, 1 out]
              n123 = call "KM_appendline.vi"("Time (s)"=w283, "temperature"=w282, "Field"=w280, "angle (deg)"=w281, "pm lorentzian"=w284, "Save frequency scan"=w285, "read/write control"=KM_file_--_read-write_control."append one line", "name or relative path"="File name") -> ()  [unwired: 12 in]
            }
            frame "Update range" {
              n124 = Unbundle By Name(w306) -> ("omega(0)"=w297:dbl, "Gamma"=w304:dbl)
              n125 = call "cursor window logic V3.vi"("cursor window action"=cursor_window_action."read", "cursor window in"=w299) -> ("cursor window out"=w302:T8)  [unwired: 8 in, 1 out]
              n126 = Unbundle By Name(w302) -> ("left"=w301:dbl, "right"=w300:dbl, "window"=w294:dbl)
              n127 = Multiply(x=w294, y=2.0 ("lower")) -> (x*y=w295:dbl)
              n128 = Multiply(x=w294, y=0.002 ("lower")) -> (x*y=w292:dbl)
              n129 = call "Q -- check range -- i -- real.vi"("upper"=w300, "lower"=w301, "number"=w297) -> ("in range?"=w305:bool)  [unwired: 6 in, 2 out]
              n130 = call "Q -- check range -- i -- real.vi"("upper"=w295, "lower"=w292, "number"=w304) -> ("in range?"=w303:bool)  [unwired: 6 in, 2 out]
              n131 = And(x=w305, y=w303) -> (x .and. y?=w298:bool)
              "fit is fine" <- w298
              n132 = case shown="True" w298 {
                tunnel: w304 -> [_ w314]
                tunnel: w297 -> [_ w315]
                tunnel: w308 -> [_ w316]
                tunnel: w307 -> [_ _]
                frame False {
                }
                frame True {
                  n133 = Compound Arithmetic op=MULTIPLY("gamma factor", w314, 2.0 ("value")) -> (w312:dbl)
                  n134 = call "cursor window logic V3.vi"("cursor window action"=cursor_window_action."change window", "window"=w312, "center"=w315, "cursor window in"=w316) -> ()  [unwired: 6 in, 2 out]
                }
              }
            }
            frame "Fit" {
              n135 = call "cursor window logic V3.vi"("cursor window action"=cursor_window_action."read", "cursor window in"=w328) -> ("cursor window out"=w324:T8)  [unwired: 8 in, 1 out]
              n136 = call "acquire cursor window data.vi"("z in"=w323, "omega in"=w326, "cursor window"=w324) -> ("z out"=w325:cdb[], "omega  out"=w327:dbl[])  [unwired: 4 in, 3 out]
              n137 = call "KM_peak -- find -- pm - V1.vi"("omega in"=w327, "z in"=w325, "parameters: complex fit"="parameters: complex fit", "plots: filter related"=w330, "plot staff ?"="plot staff", "just guess?"="use fast fit?", "subtract linear BG"=FALSE) -> ("pm lorentzian"=w322:T6)  [unwired: 10 in, 2 out]
              n138 = disable-structure shown="Disabled" {
                disable-tunnel: w322 -> [w343 _]
                disable-tunnel: w323 -> [w342 _]
                frame Disabled {
                  n139 = for {
                    tunnel: four-corner_circle_transformation."to  canonical" ("4 corner circle transformation") -> [w352]
                    tunnel: w343 -> [w351]
                    tunnel: w342 -> [w350] mode=indexing
                    tunnel: [w349] -> w341 mode=indexing
                    n140 = call "lorentzian transformations.vi"("4 corner circle transformation"=w352, "lorentzian in"=w351, "voltage in"=w350) -> ("voltage out"=w349:cdb)  [unwired: 7 in, 1 out]
                  }
                  n141 = Complex To Polar(r * e^(i*theta)=w341) -> (theta=w339:dbl[])  [unwired: 1 out]
                  n142 = Complex To Re/Im(x + iy=w341) -> (x=w346:dbl[], y=w347:dbl[])
                  n143 = Bundle(w346, w347) -> (→"Plot: frequency shift vs T 2":cluster{dbl[], dbl[]})  [unwired: 1 in]
                  n144 = Add(x=w339, y=1.5707963267948966) -> (x+y=w337:dbl[])
                  n145 = Array Size(array=w337) -> (size(s)=w338:i32)
                  n146 = for {
                    N: w338 -> [_]
                    tunnel: [w348] -> w336 mode=indexing
                    i -> [w348]
                  }
                  n147 = Bundle(w336, w337) -> (→"Plot: frequency shift vs T 3":cluster{i32[], dbl[]})  [unwired: 1 in]
                }
                frame Enabled {
                }
              }
              n148 = local write "pm lorentzian"(w322) -> ()
              n149 = Unbundle By Name(w322) -> ("omega(0)"=→"circle frequency (Hz)":dbl, "Gamma"=→"circle gamma (Hz)":dbl, "phase"=→"circle phase (rad)":dbl, "Q"=→"circle Q":dbl)
            }
            frame "Void", Default {
            }
          }
        }
      }
      event Timeout {
        n150 = event-data() -> ()  [unwired: 1 in, 2 out]
      }
    }
    n151 = Wait (ms)(milliseconds to wait=u32 0) -> ()  [unwired: 1 out]
  }
  n152 = register-events(w47) -> (reference out=w49:refnum<event-registration>)  [unwired: 2 in, 1 out]
  n153 = while {
    tunnel: w49 -> [w362]
    tunnel: w36 -> [w360]
    tunnel: w22 -> [w359]
    tunnel: w4 -> [w356]
    stop <- FALSE stop-if-true
    n154 = local read "pm lorentzian"() -> (w358:T6)
    n155 = local read "MFLI mode"() -> (w355:enum32{"circles sweep", "read", "circle PLL"})
    n156 = event shown="[2] \"center freq (Hz)\": Value Change" {
      selector: w362 -> [_ _ _ _ _ _ _ _ _]
      dyn-events: _ -> [_ _ _ _ _ _ _ _ _]
      timeout: _ -> [_ _ _ _ _ _ _ _ _]
      tunnel: w360 -> [_ w364 w385 _ w394 _ _ w425 w479]
      tunnel: [_ _ _ _ _ _ _ _ "Update system parameters"] -> _
      tunnel: w359 -> [_ w367 w384 _ _ _ _ w421 _]
      tunnel: w358 -> [_ _ _ _ _ w399 w410 _ _]
      tunnel: w356 -> [_ w365 _ _ _ _ _ w420 _]
      tunnel: [_ _ _ "refresh" _ _ _ _ _] -> _
      tunnel: w355 -> [_ w363 w383 _ _ _ _ _ _]
      event Timeout {
        n157 = event-data() -> ()  [unwired: 1 in, 2 out]
      }
      event "Plot: circle sweep window": Cursor Move {
        n158 = event-data() -> ("CursIdx"=w366:i32)  [unwired: 1 in, 8 out]
        n159 = case shown="0..2" w366 {
          selector: w366 -> [w375 w381]
          tunnel: w367 -> [w377 _]
          tunnel: w365 -> [_ w380]
          tunnel: w364 -> [w369 _]
          tunnel: w363 -> [w368 _]
          frame 0..2 {
            n160 = call "cursor window logic V3.vi"("CursIdx"=w375, "cursor window action"=cursor_window_action."cursor moves", "cursor window in"=w377) -> ("cursor window out"=w374:T8)  [unwired: 7 in, 1 out]
            n161 = Unbundle By Name(w374) -> ("left"=→"left freq (Hz)":dbl, "right"=→"right freq (Hz)":dbl, "center"=→"center freq (Hz)":dbl, "window"=→"window  (Hz)":dbl)
            n162 = case shown="\"read\", Default" w368 {
              tunnel: w369 -> [w379 _]
              frame "circles sweep" {
                w378 = "Fit"  # event data
                n163 = Generate User Event(user event=w379, event data cluster=w378) -> ()  [unwired: 2 in, 2 out]
              }
              frame "read", Default {
              }
            }
          }
          frame 3..5, Default {
            n164 = call "cursor window logic V3.vi"("CursIdx"=w381, "cursor window action"=cursor_window_action."cursor moves", "cursor window in"=w380) -> ()  [unwired: 7 in, 2 out]
          }
        }
      }
      event "center freq (Hz)": Value Change {
        n165 = event-data() -> ()  [unwired: 1 in, 6 out]
        n166 = local read "center freq (Hz)"() -> (w386:dbl)
        n167 = case shown="\"circles sweep\"" w383 {
          tunnel: w385 -> [w389 _]
          frame "circles sweep" {
            n168 = Generate User Event(user event=w389, event data cluster="Fit" ("event data")) -> ()  [unwired: 2 in, 2 out]
          }
          frame "read", Default {
          }
        }
        n169 = call "cursor window logic V3.vi"("cursor window action"=cursor_window_action."change cen&win", "center"=w386, "cursor window in"=w384) -> ()  [unwired: 7 in, 2 out]
      }
      event "refresh": Value Change {
        n170 = event-data() -> ()  [unwired: 1 in, 6 out]
        n171 = local read "reqested size"() -> (w390:i64)
        n172 = call "fucking PID.vi"("requested size"=w390, "PID action"=agregator_--_action."init") -> ()  [unwired: 9 in, 1 out]
      }
      event "Plot: circle sweep window": Cursor Release {
        n173 = event-data() -> ("CursIdx"=w393:i32)  [unwired: 1 in, 8 out]
        n174 = case shown="3, Default" w393 {
          tunnel: w394 -> [_ w395]
          frame 3, Default {
          }
          frame 0..2 {
            w396 = "Fit"  # event data
            n175 = Generate User Event(user event=w395, event data cluster=w396) -> ()  [unwired: 2 in, 2 out]
          }
        }
      }
      event "scale gauge: Plot: complex plane": Value Change {
        n176 = event-data() -> ("NewVal"=w398:dbl)  [unwired: 1 in, 5 out]
        n177 = Unbundle By Name(w399) -> ()  [unwired: 1 out]
        n178 = Unbundle By Name(w399) -> ("4corners.z center"=w400:cdb)
        n179 = control-ref of="Plot: complex plane"() -> (w397:refnum<vi>)
        n180 = Complex To Re/Im(x + iy=w400) -> (x=w401:dbl, y=w402:dbl)
        n181 = Negate(x=w398) -> (-x=w407:dbl)
        n182 = Add(x=w402, y=w407) -> (x+y=w403:dbl)
        n183 = Add(x=w401, y=w398) -> (x+y=w405:dbl)
        n184 = Add(x=w401, y=w407) -> (x+y=w406:dbl)
        n185 = Add(x=w402, y=w398) -> (x+y=w404:dbl)
        n186 = property on="Property Node" class="XYGraph (strict)"(reference=w397, "XScale.Minimum"=w406, "XScale.Maximum"=w405, "YScale.Maximum"=w404, "YScale.Minimum"=w403) -> ()  [unwired: 1 in, 2 out]
      }
      event "scale gauge: Plot: complex plane - filter": Value Change {
        n187 = event-data() -> ("NewVal"=w409:dbl)  [unwired: 1 in, 5 out]
        n188 = Unbundle By Name(w410) -> ()  [unwired: 1 out]
        n189 = Unbundle By Name(w410) -> ("4corners.z center"=w411:cdb)
        n190 = control-ref of="Plot: complex plane - filter"() -> (w408:refnum<vi>)
        n191 = Complex To Re/Im(x + iy=w411) -> (x=w412:dbl, y=w413:dbl)
        n192 = Negate(x=w409) -> (-x=w418:dbl)
        n193 = Add(x=w413, y=w418) -> (x+y=w414:dbl)
        n194 = Add(x=w412, y=w409) -> (x+y=w416:dbl)
        n195 = Add(x=w412, y=w418) -> (x+y=w417:dbl)
        n196 = Add(x=w413, y=w409) -> (x+y=w415:dbl)
        n197 = property on="Property Node" class="XYGraph (strict)"(reference=w408, "XScale.Minimum"=w417, "XScale.Maximum"=w416, "YScale.Maximum"=w415, "YScale.Minimum"=w414) -> ()  [unwired: 1 in, 2 out]
      }
      event Key Down {
        n198 = event-data() -> ("Char"=w423:i16, "VKey"=w426:T13)  [unwired: 1 in]
        "Char" <- w423
        "VKey" <- w426
        n199 = local read "MFLI mode"() -> (w419:enum32{"circles sweep", "read", "circle PLL"})
        n200 = Build Array(w423) -> (w424:i16[])
        n201 = Byte Array To String(unsigned byte array=w424) -> (string=w422:string)
        n202 = case shown="\"Up\"..\"Right\"" w426 {
          selector: w426 -> [_ _ _ _ w472]
          tunnel: w423 -> [_ _ _ _ _]
          tunnel: w425 -> [w430 _ _ _ w471]
          tunnel: w422 -> [w429 _ _ _ _]
          tunnel: w421 -> [w428 _ _ _ w464]
          tunnel: w420 -> [w427 _ _ _ _]
          tunnel: w419 -> [_ _ _ _ w463]
          frame "ASCII", Default {
            n203 = case shown="\"a\"" w429 {
              selector: w429 -> [_ _ _ w436 _ _ _]
              tunnel: w430 -> [_ _ _ _ _ _ _]
              tunnel: w428 -> [_ w431 w433 w437 w444 w447 w462]
              tunnel: w427 -> [_ _ _ _ w442 _ _]
              frame "0", Default {
              }
              frame "a" {
                n204 = call "cursor window logic V3.vi"("cursor window action"=cursor_window_action."zoom to all data", "cursor window in"=w431) -> ()  [unwired: 8 in, 2 out]
              }
              frame "?" {
                # "?"
                n205 = call "cursor window logic V3.vi"("cursor window action"=cursor_window_action."zoom X", "cursor window in"=w433) -> ()  [unwired: 8 in, 2 out]
              }
              frame "+", "-", "<", ">" {
                # "?"
                n206 = case shown="\"+\", Default" w436 {
                  tunnel: [cursor_window_action."slide right" ("cursor window action") cursor_window_action."slide left" ("cursor window action") cursor_window_action."zoom in" ("cursor window action") cursor_window_action."zoom out" ("cursor window action")] -> w435
                  frame ">" {
                  }
                  frame "<" {
                  }
                  frame "+", Default {
                  }
                  frame "-" {
                  }
                }
                n207 = call "cursor window logic V3.vi"("cursor window action"=w435, "cursor window in"=w437) -> ()  [unwired: 8 in, 2 out]
              }
              frame "c" {
                n208 = call "cursor window logic V3.vi"("cursor window action"=cursor_window_action."check", "cursor window in"=w444) -> ()  [unwired: 8 in, 2 out]
                n209 = call "cursor window logic V3.vi"("cursor window action"=cursor_window_action."check", "cursor window in"=w442) -> ()  [unwired: 8 in, 2 out]
              }
              frame "t" {
                n210 = local read "talk to MFLI !"() -> (w446:bool)
                n211 = case shown="True" w446 {
                  tunnel: w447 -> [_ w453]
                  frame False {
                  }
                  frame True {
                    n212 = local read "Auto-update sweep window!"() -> (w452:bool)
                    n213 = Not(x=w452) -> (.not. x?=w451:bool)
                    n214 = local write "Auto-update sweep window!"(w451) -> ()
                    n215 = Select(t=cursor_window_action."color--green" ("cursor window action"), s=w451, f=cursor_window_action."color--red" ("cursor window action")) -> (s? t:f=w448:T15)
                    n216 = call "cursor window logic V3.vi"("cursor window action"=w448, "cursor window in"=w453) -> ()  [unwired: 8 in, 2 out]
                  }
                }
              }
              frame "r" {
                n217 = local read "Auto-update sweep window!"() -> (w457:bool)
                n218 = local read "talk to MFLI !"() -> (w458:bool)
                n219 = Not(x=w458) -> (.not. x?=w461:bool)
                n220 = Select(t=cursor_window_action."color--green" ("cursor window action"), s=w457, f=cursor_window_action."color--red" ("cursor window action")) -> (s? t:f=w454:T15)
                n221 = Select(t=w454, s=w461, f=cursor_window_action."color--yellow" ("cursor window action")) -> (s? t:f=w459:T15)
                n222 = local write "talk to MFLI !"(w461) -> ()
                n223 = call "cursor window logic V3.vi"("cursor window action"=w459, "cursor window in"=w462) -> ()  [unwired: 8 in, 2 out]
              }
            }
          }
          frame "Escape" {
          }
          frame "PageUp" {
          }
          frame "PageDown" {
          }
          frame "Up".."Right" {
            n224 = case shown="\"Left\"" w472 {
              tunnel: [cursor_window_action."move right" ("cursor window action") cursor_window_action."move left" ("cursor window action") cursor_window_action."broaden" ("cursor window action") cursor_window_action."shrink" ("cursor window action")] -> w466
              frame "Right", Default {
              }
              frame "Left" {
              }
              frame "Up" {
              }
              frame "Down" {
              }
            }
            n225 = call "cursor window logic V3.vi"("cursor window action"=w466, "cursor window in"=w464) -> ("cursor window out"=w465:T8)  [unwired: 8 in, 1 out]
            n226 = Unbundle By Name(w465) -> ("left"=w470:dbl, "right"=w469:dbl, "center"=w468:dbl, "window"=w467:dbl)
            n227 = case shown="\"circles sweep\"" w463 {
              tunnel: w471 -> [w474 _]
              frame "circles sweep" {
                w473 = "Fit"  # event data
                n228 = Generate User Event(user event=w474, event data cluster=w473) -> ()  [unwired: 2 in, 2 out]
              }
              frame "read", Default {
              }
            }
            n229 = local write "window  (Hz)"(w467) -> ()
            n230 = local write "right freq (Hz)"(w469) -> ()
            n231 = local write "center freq (Hz)"(w468) -> ()
            n232 = local write "left freq (Hz)"(w470) -> ()
          }
        }
      }
      event "Update system parameters": Value Change {
        n233 = event-data() -> ()  [unwired: 1 in, 6 out]
        n234 = Generate User Event(user event=w479, event data cluster="Update system parameters" ("event data")) -> ()  [unwired: 2 in, 2 out]
      }
    }
    n235 = Wait (ms)(milliseconds to wait=u32 0) -> ()  [unwired: 1 out]
  }
